vi "cRIO_4DOF_Admittance_control_v8c_eightmaze_MESO_removeIR.vi"() -> ()   [LabVIEW 2019]
uses:
  <vilib>/Platform/TimedLoop/XDataNode/timing_clust.ctl
  <vilib>/Platform/TimedLoop/XDataNode/nitl_modes.ctl
  <vilib>/Platform/TimedLoop/XDataNode/wakeup.ctl
  <vilib>/Analysis/baseanly.llb/Mean (DBL).vi
  Global 1.vi
  <vilib>/imath/engines/lvmath2/RunTimeEngine/NodeEndStatement/NIMS_NodeEndStatement_Output.vi
  <instcachedir>/0/NIMS_NodeEndStatement_Output_53EC0D466D134D7ABD903AC30B43404B.lvgen/NIMS_NodeEndStatement_Output_53EC0D466D134D7ABD903AC30B43404B_001.vi
  <vilib>/imath/engines/lvmath2/RunTimeEngine/ErrorHandling/NIMS_Finalize Error.vi
  <vilib>/imath/engines/lvmath2/RunTimeEngine/IndexReplace/NIMS V(S)=S.vi
  <instcachedir>/0/NIMS V(S)=S_BD5C8CB81B6E4D99B8C0034EA1BEE55D.lvgen/NIMS V(S)=S_BD5C8CB81B6E4D99B8C0034EA1BEE55D_000.vi
  <vilib>/imathl/engines/lvmath/Functions/Error Handling/Create Error.vi
  <instcachedir>/0/NIMS_NodeEndStatement_Output_53EC0D466D134D7ABD903AC30B43404B.lvgen/NIMS_NodeEndStatement_Output_53EC0D466D134D7ABD903AC30B43404B_005.vi
  <vilib>/addons/control/pid/pid.llb/PID (DBL Array).vi
  <vilib>/imath/engines/lvmath2/RunTimeEngine/ArithmeticOperatorToken/NIMS_ArithmeticOperator_multmx(M,CV).vi
  <instcachedir>/0/NIMS_ArithmeticOperator_multmx(M,CV)_1D61EED49E1847F3B05DBB8EDD2FBF8F.lvgen/NIMS_ArithmeticOperator_multmx(M,CV)_1D61EED49E1847F3B05DBB8EDD2FBF8F_000.vi
  <instcachedir>/0/NIMS_NodeEndStatement_Output_53EC0D466D134D7ABD903AC30B43404B.lvgen/NIMS_NodeEndStatement_Output_53EC0D466D134D7ABD903AC30B43404B_002.vi
  <vilib>/imath/engines/lvmath2/RunTimeEngine/BuiltInFunctions/inv/NIMS_inv(GM).vi
  <instcachedir>/0/NIMS_inv(GM)_A6DF8FE880224208AACFE4CF9F659502.lvgen/NIMS_inv(GM)_A6DF8FE880224208AACFE4CF9F659502_000.vi
  <vilib>/imath/engines/lvmath2/RunTimeEngine/ErrorHandling/NIMS_Create Error From Enums.vi
  <vilib>/imath/engines/lvmath2/RunTimeEngine/IndexRead/NIMS M(R2,S).vi
  <instcachedir>/0/NIMS M(R2,S)_56813DCFDD5A484292D2195AF15D2BF5.lvgen/NIMS M(R2,S)_56813DCFDD5A484292D2195AF15D2BF5_000.vi
  <vilib>/imath/engines/lvmath2/RunTimeEngine/IndexRead/NIMS M(S,S).vi
  <instcachedir>/0/NIMS M(S,S)_AC51E74150A542F7991B9634C66F3096.lvgen/NIMS M(S,S)_AC51E74150A542F7991B9634C66F3096_000.vi
  <vilib>/imath/engines/lvmath2/RunTimeEngine/Managers/WorkSpace/UID Generator.vi
  <vilib>/imath/engines/lvmath2/RunTimeEngine/BuiltInFunctions/round/NIMS_round(DBL-S).vi
  <vilib>/imath/engines/lvmath2/RunTimeEngine/IndexRead/NIMS V(S).vi
  <instcachedir>/0/NIMS V(S)_0488751826AF41519A22953C041130DC.lvgen/NIMS V(S)_0488751826AF41519A22953C041130DC_000.vi
  <vilib>/imath/engines/lvmath2/RunTimeEngine/RunTimeType/NIMS_RunTimeType_From StrictType (excl LVString).vi
  <instcachedir>/0/NIMS_RunTimeType_From StrictType (excl LVString)_D8AFBA86A94845AAA577C895450664BD.lvgen/NIMS_RunTimeType_From StrictType (excl LVString)_D8AFBA86A94845AAA577C895450664BD_000.vi
  <vilib>/imath/engines/lvmath2/RunTimeEngine/LocalVariableDefStatement/MC_LocalVariableDefStatement_Display.vi
  <vilib>/imath/engines/lvmath2/RunTimeEngine/BuiltInFunctions/all/NIMS_all(GS).vi
  <vilib>/imath/engines/lvmath2/RunTimeEngine/Managers/SymbolTable/Clear UID.vi
  <vilib>/imath/engines/lvmath2/RunTimeEngine/ArithmeticOperatorToken/NIMS_ArithmeticOperator_power(S).vi
  <instcachedir>/0/NIMS_ArithmeticOperator_power(S)_F1497A2DE3CE4E82B2C3646D59904248.lvgen/NIMS_ArithmeticOperator_power(S)_F1497A2DE3CE4E82B2C3646D59904248_014.vi
  <vilib>/imath/engines/lvmath2/RunTimeEngine/BuiltInFunctions/cross/NIMS_cross(GV,GV).vi
  <instcachedir>/0/NIMS_cross(GV,GV)_6F1F1C643EFF41C8A983D972A94A5A15.lvgen/NIMS_cross(GV,GV)_6F1F1C643EFF41C8A983D972A94A5A15_000.vi
  <vilib>/imath/engines/lvmath2/RunTimeEngine/IndexRead/NIMS M(S).vi
  <instcachedir>/0/NIMS M(S)_B826C018497E4940AE96BD27B540B6FB.lvgen/NIMS M(S)_B826C018497E4940AE96BD27B540B6FB_000.vi
  <vilib>/imath/engines/lvmath2/RunTimeEngine/BuiltInFunctions/norm/NIMS_norm(GM,DBL).vi
  <instcachedir>/0/NIMS_norm(GM,DBL)_8BCB088F207E48DF95CF5C1DC502F84D.lvgen/NIMS_norm(GM,DBL)_8BCB088F207E48DF95CF5C1DC502F84D_000.vi
  <vilib>/imath/engines/lvmath2/RunTimeEngine/BuiltInFunctions/norm/NIMS_norm(GV,DBL).vi
  <instcachedir>/0/NIMS_norm(GV,DBL)_4A8B6F23BC0A47549B8AB805006257D9.lvgen/NIMS_norm(GV,DBL)_4A8B6F23BC0A47549B8AB805006257D9_000.vi
  <vilib>/imath/engines/lvmath2/RunTimeEngine/BuiltInFunctions/dot/NIMS_dot(GM,GM,12).vi
  <instcachedir>/0/NIMS_dot(GM,GM,12)_05F0B1C82C6743E4843530F9B3085698.lvgen/NIMS_dot(GM,GM,12)_05F0B1C82C6743E4843530F9B3085698_000.vi
  <vilib>/imath/engines/lvmath2/RunTimeEngine/ArithmeticOperatorToken/NIMS_ArithmeticOperator_minus.vi
  <instcachedir>/0/NIMS_ArithmeticOperator_minus_12BFF9710EA5430A9EE87C5BC3F65186.lvgen/NIMS_ArithmeticOperator_minus_12BFF9710EA5430A9EE87C5BC3F65186_003.vi
  <vilib>/platform/TimedLoop/XDataNode/XDataNode.xnode
  <resource>/objmgr/ni.dex.rc
  <vilib>/addons/control/pid/NI_PID_pid.lvlib
  <vilib>/Analysis/NI_AALBase.lvlib
  <vilib>/Platform/TimedLoop/XDataNode/XDNodeRunTimeDep.lvlib
  <vilib>/imath/engines/lvmath2/RunTimeEngine/Managers/SymbolTable/NIMS_WorkSpace.lvlib
panel:
  in  "Global offset":dbl[](array[numeric])=[0.0, 0.0, 0.0, 0.0]
  in  "Half Dzone Limit":bool=TRUE
  in  "servo wait (ms)":u32=800
  in  "Servo enable":bool
  in  "No LEDs":bool=TRUE
  in  "Manual \npulse high":bool
  in  "cx start":dbl=1.0 format="%#_13g"
  in  "LED_R 2":bool
  in  "LED_L 2":bool
  in  "Flash LEDs":bool
  out "SynPulseOn":bool
  in  "RunOnceLatch":bool
  out "Data syncing":bool
  in  "No LED no Sound":bool
  in  "Mouse YStop":dbl=-0.33 format="%#_13g"
  out "Rmag":dbl
  out "w_cen 2":dbl[](array[numeric])
  out "Eight maze on":bool
  out "Loop_R Exit":bool
  out "Loop_L Exit":bool
  out "exit_pos":dbl[](array[numeric])
  out "Rexit":dbl
  out "exit_cen":dbl[](array[numeric])
  in  "End Wheel":bool
  in  "w_cen":dbl[](array[numeric])=[0.06, -0.2]
  in  "Rwheel":dbl=0.06
  in  "Begin Wheel":bool
  in  "delpos limits (+/-)\nadmittance control \nLoop":dbl[](array[numeric])=[0.0012, 0.0002, 0.0, 0.01]
  in  "delpos limits (+/-)\nadmittance control \nDzone":dbl[](array[numeric])=[0.0008, 0.0002, 0.0, 0.01]
  in  "Lego2":dbl=-0.03
  in  "Lego1":dbl=0.07
  in  "Ftrans":bool=TRUE
  out "TransF":dbl[](array[numeric])
  in  "d_{1}_{2} (mm)":dbl[](array[numeric])=[10.0, 0.0, 0.0]
  in  "MDsRy":dbl=0.251
  in  "MDsLy":dbl=-0.251
  out "MDsetup":bool
  in  "MDpos_lims":dbl[](array[numeric])=[0.0005, 0.0005]
  in  "MDstopR":dbl=0.025
  in  "Disable X":bool
  in  "MDstopL":dbl=0.023
  in  "Disable -X Dzone":bool
  in  "PWMset2":dbl[](array[numeric])=[8.1, 5.2, 5.45]
  in  "PWMset1":dbl[](array[numeric])=[3.4, 5.2, 5.45]
  in  "cMD":dbl=0.3 format="%#_13g"
  in  "mMD":dbl=0.02 format="%#_13g"
  in  "MDzone":dbl[](array[numeric])=[0.04, 0.027]
  out "Rsmall":dbl
  in  "Loop radius":dbl=0.127 format="%#_13g"
  in  "PWM positions":dbl[](array[numeric])=[4.5, 3.4, 5.1, 5.8]
  in  "PWM rate":dbl[](array[numeric])=[0.1, 0.1, 0.1, 0.1]
  out "appended array":bool[](array[boolean])
  in  "LED_L":bool
  in  "LED_R":bool
  in  "MD_L":bool
  in  "MD_R":bool
  out "Left":bool=TRUE
  in  "AIR":bool
  in  "Sound":bool
  out "Right":bool=TRUE
  in  "MD time (ms)":i32=4000
  in  "Loop seq.":dbl
  in  "Initialize":bool=TRUE
  in  "No Milk":bool
  out "All BBL":bool
  out "BB3_L":bool
  out "BB2_L":bool
  out "BB1_R":bool
  out "All BBR":bool
  out "BB3_R":bool
  out "BB2_R":bool
  out "BB1_L":bool
  out "Seq update":i32
  in  "Repeat sound":bool
  in  "Air puff time":u32=1000
  out "Direction array":bool[](array[boolean])=[TRUE, FALSE, FALSE, TRUE, FALSE, TRUE, TRUE, FALSE, TRUE, FALSE, FALSE, TRUE, FALSE, TRUE, FALSE, FALSE, TRUE, FALSE, TRUE, TRUE, FALSE, TRUE, FALSE, FALSE, TRUE, FALSE, TRUE, TRUE, FALSE, TRUE, FALSE, FALSE, TRUE, FALSE, TRUE, TRUE, FALSE, TRUE, FALSE, FALSE, TRUE, FALSE, TRUE, TRUE, FALSE, TRUE, FALSE, FALSE, TRUE]
  in  "cTrans":dbl=0.01 format="%#_13g"
  out "C":dbl
  out "Dzone y 2":dbl=-0.0607 format="%#_13g"
  in  "Vector correction":bool=TRUE
  in  "manual homing stop":bool
  in  "cLoop":dbl=0.3
  in  "mLoop":dbl=0.02
  out "c_applied":dbl[][](array[numeric])
  out "m_applied":dbl[][](array[numeric])
  in  "lower Z limit":dbl=-0.782
  out "Jostick offset":dbl[](array[numeric])
  out "Pos":dbl[](array[numeric])
  out "targetpos":dbl[](array[numeric])
  out "Rotz":dbl[][](array[numeric])
  in  "Eight maze on":bool
  out "Gradient R":dbl=0.0293 format="%#_13g"
  out "Radius":dbl=0.0293 format="%#_13g"
  out "Dzone y":dbl=0.025 format="%#_13g"
  out "Loop_L":bool
  out "F":dbl[](array[numeric])
  in  "number Fsamples":i32=10
  out "Homed":bool[](array[boolean])
  out "Hall voltages":dbl[](array[numeric])
  in  "Joint offset":dbl[](array[numeric])
  in  "Target HallV":dbl[](array[numeric])=[0.1, 0.1, 0.1]
  out "Raw voltages":dbl[](array[numeric])
  in  "Record to current file":bool
  in  "Close file and open new file":bool
  in  "Stop raspberry pi":bool
  out "changes from \nadmittance {m}":dbl[](array[numeric])
  out "Joystick input":dbl[](array[numeric])
  in  "Joystick control on":bool
  out "Z position":T1(graph)
  out "Loop_R":bool
  out "Trajectory changes in Yaw":T1(graph)
  in  "Mouse force limits":dbl[](array[numeric])=[0.5, 0.2, 0.0, 0.025]
  out "loop":i32
  in  "Disable Yaw forces":bool=TRUE
  in  "Admittance scale":dbl[](array[numeric])=[1.0, 1.0, 0.0, 1.0]
  out "velocity \n(mouseframe)":dbl[](array[numeric])
  in  "RETURN TO HOME \nPOSITION AND STOP":bool
  out "Dzone":bool
  in  "deltapos":dbl[](array[numeric]) format="%#_13g"
  in  "delpos limits (+/-) \ntrajectory control\n(global frame)":dbl[](array[numeric])=[0.002, 0.002, 0.0, 0.02]
  in  "delpos limits (+/-)\nadmittance control \n(mouse frame)":dbl[](array[numeric])=[0.0015, 0.0002, 0.0, 0.01]
  in  "lower limit":dbl[](array[numeric])=[-0.3, -0.34, -0.782, -6000.0]
  in  "upper limit":dbl[](array[numeric])=[0.3, 0.18, -0.65, 6000.0]
  out "Dzone x":dbl=-0.0607 format="%#_13g"
  in  "Trajectory scale":dbl[](array[numeric])=[0.05, 0.05, 0.0, 0.05]
  out "Trajectory changes in XY":T1(graph)
  in  "Disable Y forces":bool=TRUE
  out "changes from trajectory":dbl[](array[numeric])
  in  "Y_trajectory":bool
  in  "Disable -X":bool=TRUE
  out "Eightmaze_switch":bool
  in  "Yaw":dbl(slide) scale=0.0..3.142
  in  "Z":dbl(slide)=-0.7034810126582278 scale=-0.1..0.1
  in  "Y":dbl(slide)=0.05 scale=-0.29..0.05
  in  "X":dbl(slide) scale=0.0..0.06
  in  "Yaw_tajectory":bool
  out "target position":dbl[](array[numeric])
  in  "Fsense deadband\n (Nm or N)":dbl[](array[numeric])=[0.025, 0.025, 0.025, 0.001]
  in  "Output range (PWM)":cluster{"output high":dbl, "output low":dbl}[](array[cluster])=[{"output high"=100.0, "output low"=-100.0}] {"output low" format="%.2f"; "output high" format="%.2f"}
  in  "Admittance PID gains":T2(array[cluster])=[{"proportional gain (Kc)"=1.0, "integral time (Ti, min)"=0.01, "derivative time (Td, min)"=0.0}] {"derivative time (Td, min)" format="%.3f"; "integral time (Ti, min)" format="%.3f"; "proportional gain (Kc)" format="%.3f"}
  in  "Manual force":bool
  in  "Manual forces\n(mouse frame)":dbl[](array[numeric])=[0.0, 0.0, 0.0, 0.0, 0.0, 0.0]
  in  "goniometer PWM\n offset":dbl=50.0
  in  "delta PWM offset":dbl[](array[numeric])=[50.0, 50.0, 50.0]
  in  "manual position\n(global frame)":dbl[](array[numeric])=[0.0, 0.0, 0.0, 0.0, 0.0, 0.0]
  in  "Manual position control":bool
  out "Forces (N) 2":T3(graph)
  out "Torques (Nm) 2":T3(graph)
  in  "Measure Fsensor \nV offset":bool
  out "Sensor V offset":dbl[](array[numeric])
  out "Mouse forces":dbl[](array[numeric])
  in  "Out of range":bool
  out "F_measured":dbl[](array[numeric])
  out "velocity\n(global frame)":dbl[](array[numeric])
  out "Admittance changes in Yaw":T3(graph)
  out "Admittance changes in XY":T3(graph)
  out "Torques (Nm)":T3(graph)
  out "Forces (N)":T3(graph)
  in  "m":dbl[][](array[numeric])=[[0.02, 0.0, 0.0, 0.0], [0.0, 0.02, 0.0, 0.0], [0.0, 0.0, 0.30000000000000004, 0.0], [0.0, 0.0, 0.0, 2e-05]]
  in  "c":dbl[][](array[numeric])=[[0.5, 0.0, 0.0, 0.0], [0.0, 0.2, 0.0, 0.0], [0.0, 0.0, 2.0, 0.0], [0.0, 0.0, 0.0, 0.0002]]
  out "True loop time (ms)":u32
  in  "theta6":dbl
  in  "theta1,2,3 pos2":dbl=-0.75
  in  "Initial pos 2":bool
  in  "Theta PID gains":T2(array[cluster])=[{"proportional gain (Kc)"=1.0, "integral time (Ti, min)"=0.01, "derivative time (Td, min)"=0.0}] {"derivative time (Td, min)" format="%.3f"; "integral time (Ti, min)" format="%.3f"; "proportional gain (Kc)" format="%.3f"}
  in  "Theta output range":cluster{"output high":dbl, "output low":dbl}[](array[cluster])=[{"output high"=100.0, "output low"=-100.0}] {"output low" format="%.2f"; "output high" format="%.2f"}
  in  "theta 6":dbl
  in  "theta1,2,3":dbl=-0.75
  in  "Stop Joint space control":bool
  in  "Disable PID":bool
  out "velocity \n(joint space)":dbl[](array[numeric])
  out "op-space pos\n(global frame)":dbl[](array[numeric])
  out "alpha beta gamma":T1(graph)
  out "PWM":T4(graph)
  out "XY position":T1(graph)
  out "discriminant (>0)":dbl
  in  "Loop time (ms)":i64=10
  out "Data output":dbl[][](array[numeric])
  out "network stream":errorcluster
  out "Available Elements for Writing in network stream":i32
  in  "STOP saving data set":bool
  in  "PAUSE ms to wait":u32=5000
  in  "PAUSE saving data set":bool
  in  "BEGIN saving new data set":bool
  out "J":dbl[][](array[numeric])
  out "Joint_pos (rad)":dbl[](array[numeric])
  # "VALUE USED FOR INITIALISATION, TROUBLESHOOTING AND ANALYSIS"
  # "Must start USB6211DAQ.vi to read voltages from force sensor"
  # "Data saving. 'Write data to tdms file (PC VI).vi' must be started\n BEFORE this vi in order for the network stream to open correctly.\nMake sure 'Write data to tdms file (PC VI).vi' is configured correctly"
  # "Initialise system; both buttons must be pressed sequentially, left then right. Press Stop JSC when AB offset = Joint_pos"
  # "STOP AND RETURN TO HOME"
  # "VELOCITY LIMITS NB: delpos*100 = max velocity"
  # "Trajectory control. Push these buttons after manually moving the headstage to X,Y=0 m, yaw = 3.142 rad"
  # "Use Manual position control to set up or adjust the headstage position; the sliders ADD ON to the current position."
  # "POSITION LIMITS"
  # "NB: if True loop time does not equal Loop time\nthen the virtual admittance will not be correct"
  # "Admittance control. Manual position control must be switched OFF for Admittance control to work."
  # "Trajectory parameters"
  # "8 maze controls - air puff manually activated; 3000ms MD time = 8uL milk"
  # "IR camera control: record should \nremain on while recording; close \nfile and open new for each mouse"
  # "Rdown"
  # "Lup"
  # "Rup"
  # "Ldown"
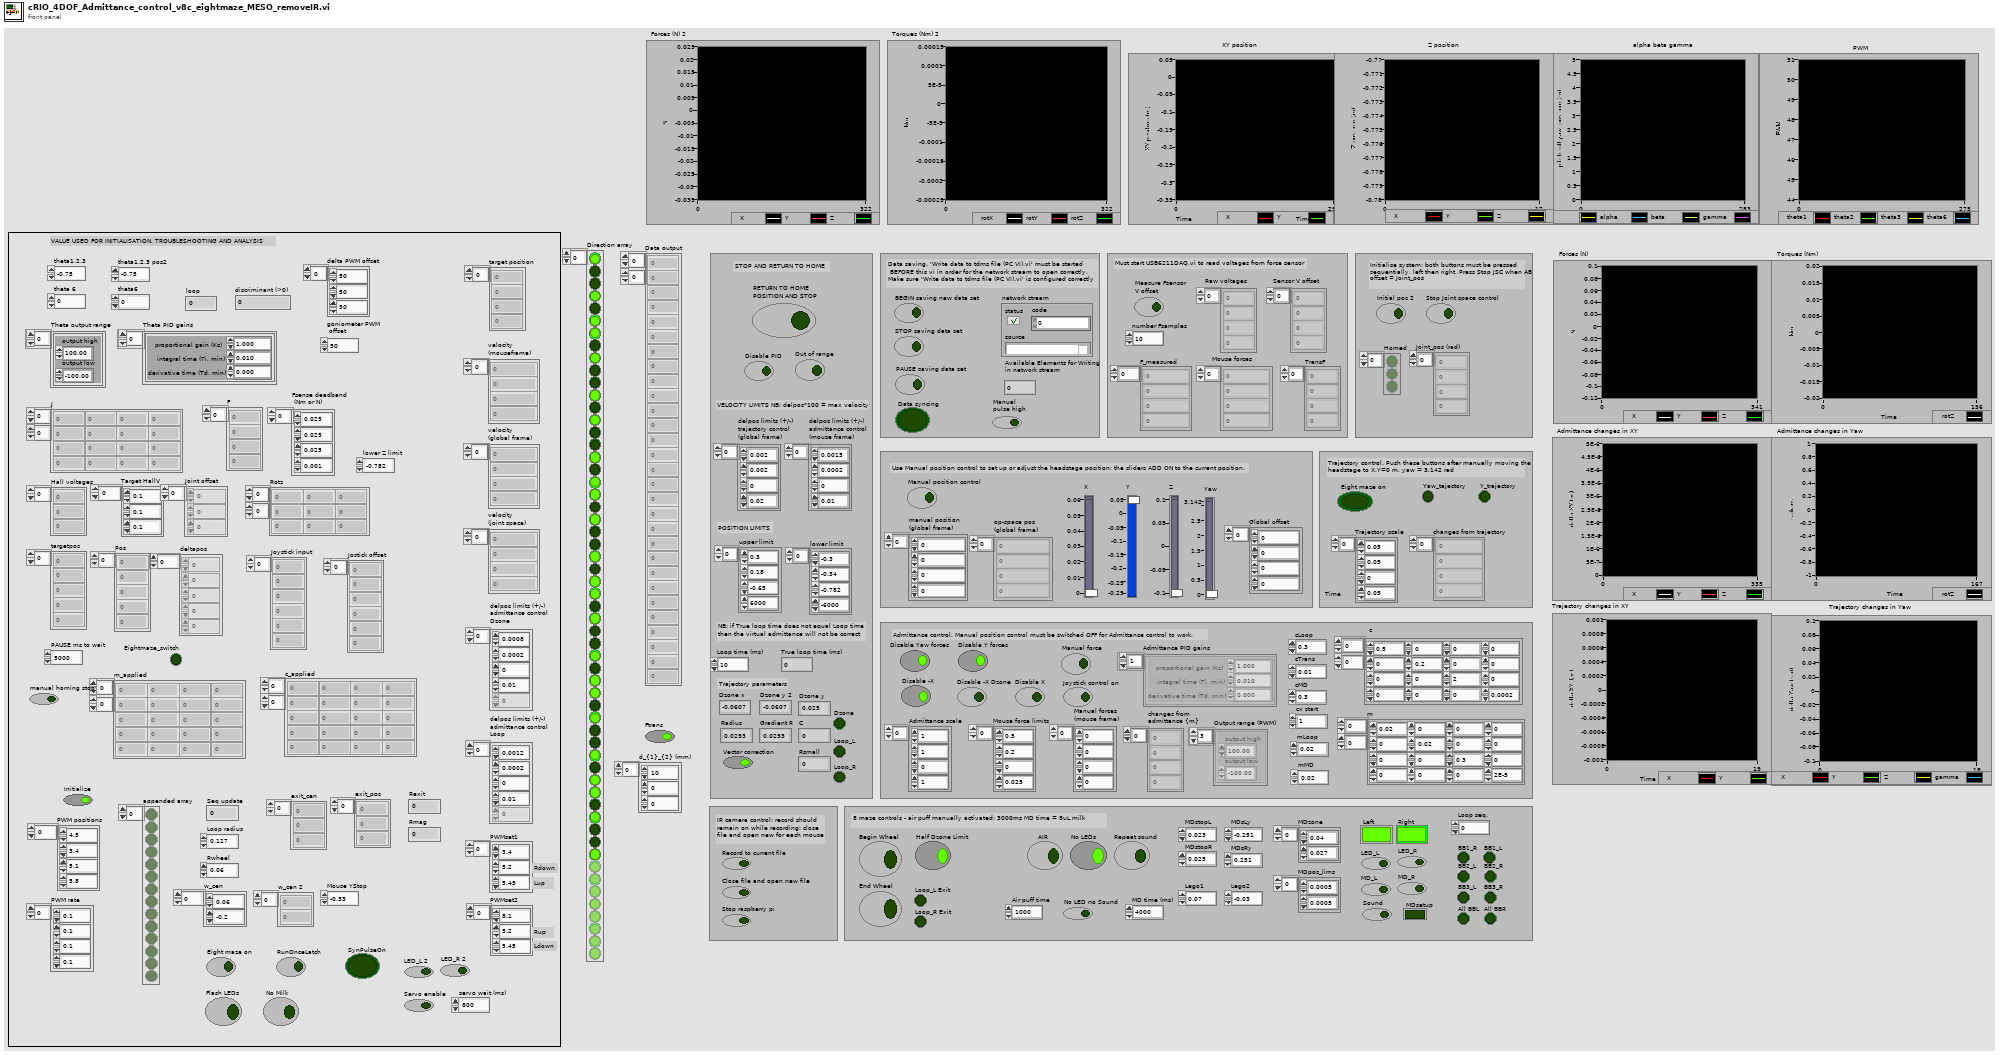
[diagram p1: front panel]
types:
  T1 = cluster{"Joint_pos (rad)[0]":dbl, "Joint_pos (rad)[1]":dbl, "Joint_pos (rad)[2]":dbl, "Joint_pos (rad)[3]":dbl, "Joint_pos (rad)[4]":dbl, "Joint_pos (rad)[5]":dbl, "Joint_pos (rad)[6]":dbl, "Joint_pos (rad)[7]":dbl, "Joint_pos (rad)[8]":dbl}
  T2 = cluster{"proportional gain (Kc)":dbl, "integral time (Ti, min)":dbl, "derivative time (Td, min)":dbl}[]
  T3 = cluster{"F[0]":dbl, "F[1]":dbl, "F[2]":dbl, "F[3]":dbl, "F[4]":dbl, "F[5]":dbl, "F[6]":dbl, "F[7]":dbl, "F[8]":dbl}
  T4 = cluster{"[0]":dbl, "[1]":dbl, "[2]":dbl, "[3]":dbl, "[4]":dbl, "[5]":dbl, "[6]":dbl, "[7]":dbl, "[8]":dbl}
  T5 = typedef "XDNodeRunTimeDep.lvlib/timing_clust.ctl" = cluster{"Expected End [f-1]":u64, "Actual End [f-1]":u64, "Finished Late? [f-1]":bool, "Expected End [i-1]":u64, "Actual End [i-1]":u64, "Finished Late? [i-1]":bool, "Expected Start [i]":u64, "Actual Start [i]":u64, "Expected Start [f]":u64, "Actual Start [f]":u64, "Source Name":string, "Structure Name":string, "Period":i64, "Deadline":i64, "Offset":i64, "Start":i64, "Priority":i32, "Timeout":i32, "Mode":T6, "Wakeup Reason":T7, "Error":errorcluster, "Source Type":string, "Secondary Source Type":string, "Global End Time":u64, "Global Start Time":u64, "Frame Duration":u64, "Iteration Duration":u64, "Assigned CPU":i32, "I/O Scan Engine Mode":u32}
  T6 = typedef "XDNodeRunTimeDep.lvlib/nitl_modes.ctl" = enum32{"No Change", "Process missed periods, maintain original phase", "Discard missed periods, maintain original phase", "Process missed periods, ignore original phase", "Discard missed periods, ignore original phase"}
  T7 = typedef "XDNodeRunTimeDep.lvlib/wakeup.ctl" = enum32{"Normal", "Aborted", "Asynchronous wakeup", "Timing source error", "Timed loop error", "Timeout"}
  T8 = cluster{"op-space pos\n(global frame)[0]":dbl, "op-space pos\n(global frame)[1]":dbl, "op-space pos\n(global frame)[2]":dbl, "op-space pos\n(global frame)[3]":dbl, "op-space pos\n(global frame)[4]":dbl, "op-space pos\n(global frame)[5]":dbl, "op-space pos\n(global frame)[6]":dbl, "op-space pos\n(global frame)[7]":dbl, "op-space pos\n(global frame)[8]":dbl}
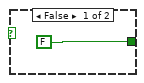
[diagram p3: hidden frame]
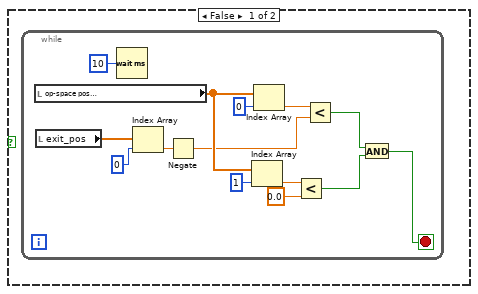
[diagram p4: hidden frame]
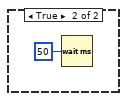
[diagram p5: hidden frame]
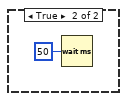
[diagram p6: hidden frame]
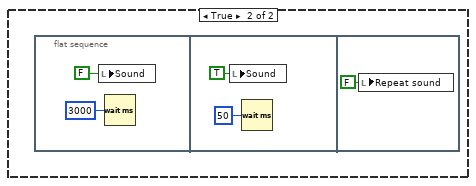
[diagram p8: hidden frame]
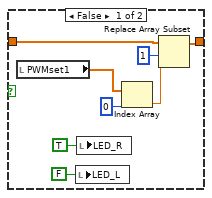
[diagram p9: hidden frame]
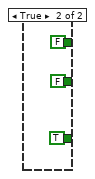
[diagram p12: hidden frame]
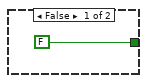
[diagram p14: hidden frame]
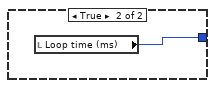
[diagram p16: hidden frame]
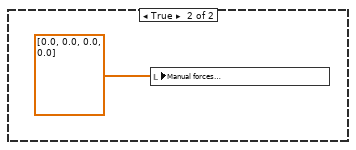
[diagram p17: hidden frame]
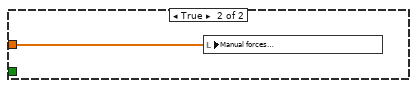
[diagram p18: hidden frame]
diagram:
  n1 = flat-sequence {
    frame #0 {
      n2 = local write "RunOnceLatch"(TRUE ("RunOnceLatch")) -> ()
    }
    frame #1 {
      n3 = while {
        stop <- FALSE stop-if-true
        n4 = flat-sequence {
          frame #0 {
            n5 = while {
              stop <- w10 stop-if-true
              n6 = local read "Eight maze on"() -> (w9:bool)
              n7 = local read "Begin Wheel"() -> (w7:bool)
              n8 = Not(x=w9) -> (.not. x?=w8:bool)
              n9 = Wait (ms)(milliseconds to wait=u32 250) -> ()  [unwired: 1 out]
              n10 = Compound Arithmetic op=AND(w7, w8, "RunOnceLatch") -> (w10:bool)
            }
          }
          frame #1 {
            n11 = disable-structure shown="Disabled" {
              frame Disabled {
                n12 = while {
                  stop <- w14 stop-if-true
                  n13 = local read "op-space pos\n(global frame)"() -> (w24:dbl[])
                  n14 = Wait (ms)(milliseconds to wait=u32 10) -> ()  [unwired: 1 out]
                  n15 = local read "w_cen"() -> (w21:dbl[])
                  n16 = Index Array(array=w21, index=0) -> (element=w19:dbl)
                  n17 = Index Array(array=w21, index=1) -> (element=w17:dbl)
                  n18 = Index Array(array=w24, index=0) -> (element=w20:dbl)
                  n19 = Index Array(array=w24, index=1) -> (element=w18:dbl)
                  n20 = local read "op-space pos\n(global frame)"() -> (w28:dbl[])
                  n21 = mathscript code="xpos = Pos(1,1);\nypos = Pos(1,2);\nzpos = Pos(1,3);\nyawpos = Pos(1,4);\n\nRotz = [cos(yawpos),-sin(yawpos),0; sin(yawpos),cos(yawpos),0; 0,0,1];\nxhat = [1, 0, 0]';\nzhat = [0, 0, 1]';\n\n       xcen = xpos - w_cen(1);\n       ycen = ypos - w_cen(2);\n       Rmag = real((xcen^2 + ycen^2)^0.5);\n       xtarg = Rwheel/Rmag*xcen  + w_cen(1);\n       ytarg = Rwheel/Rmag*ycen + w_cen(2);      \n       RLsgn = 1;\n\nvecpos = [xcen, ycen, 0]';         % position vector, zero'd circle\nvecyaw = RLsgn*cross(vecpos,zhat);  % yaw vector\nvecyaw_o = Rotz'*vecyaw;        %  yaw vector transformed by actual yaw\nyawerrsign = sign(0 - vecyaw_o(2));  % sign of yaw error\nyawerrmag = acos(dot(vecyaw_o,xhat)/(norm(vecyaw_o)*norm(xhat))); % magnitude of yaw error   \nyawtarg  = yawpos - yawerrsign*real(yawerrmag); % target yaw position\n\ntargetpos = [xtarg, ytarg, zpos, yawtarg];\n\ndelpos = real(targetpos - Pos);"("Pos"=w28, "Rwheel"="Rwheel", "w_cen"="w_cen") -> ("delpos"=w12:dbl[])  [unwired: 1 in, 1 out]
                  n22 = Less?(x=w20, y=w19) -> (x < y?=w16:bool)
                  n23 = Greater?(x=w18, y=w17) -> (0:w15:bool)
                  n24 = And(x=w16, y=w15) -> (x .and. y?=w14:bool)
                  n25 = local write "deltapos"(w12) -> ()
                }
              }
              frame Enabled {
              }
            }
          }
          frame #2 {
            n26 = local read "op-space pos\n(global frame)"() -> (w441:dbl[])
            n27 = Index Array(array=w441, index=3) -> (element=w442:dbl)
            n28 = while {
              tunnel: w442 -> [w457]
              stop <- w450 stop-if-true
              n29 = local read "op-space pos\n(global frame)"() -> (w456:dbl[])
              n30 = local read "w_cen"() -> (w455:dbl[])
              n31 = local write "Disable Yaw forces"(TRUE ("Disable Yaw forces")) -> ()
              n32 = local write "Disable Y forces"(TRUE ("Disable Y forces")) -> ()
              n33 = mathscript code="xpos = Pos(1,1);\nypos = Pos(1,2);\nzpos = Pos(1,3);\nyawpos = Pos(1,4);\n\nxtarg = 0;\nyawtarg = pi/2;\n\ntargetpos = [xtarg, ypos, zpos, yawtarg];\n\ndelpos = real(targetpos - Pos);"("yaw_init"=w457, "Pos"=w456, "w_cen"=w455) -> ("delpos"=w449:dbl[])  [unwired: 1 in, 1 out]
              n34 = local write "Disable -X"(TRUE ("Disable -X")) -> ()
              n35 = local write "delpos limits (+/-)\nadmittance control \n(mouse frame)"(dbl[] [0.0008, 0.0002, 0.0, 0.01] ("delpos limits (+/-)\nadmittance control \nDzone")) -> ()
              n36 = local read "op-space pos\n(global frame)"() -> (w453:dbl[])
              n37 = Index Array(array=w453, index=1) -> (element=w452:dbl)
              n38 = local write "deltapos"(w449) -> ()
              n39 = Greater?(x=w452, y=0.0) -> (0:w450:bool)
              n40 = Wait (ms)(milliseconds to wait=u32 10) -> ()  [unwired: 1 out]
            }
          }
          frame #3 {
            n41 = local write "RunOnceLatch"(FALSE ("RunOnceLatch")) -> ()
            n42 = local write "Eight maze on"(TRUE ("Eight maze on")) -> ()
            n43 = local write "Begin Wheel"(FALSE ("Begin Wheel")) -> ()
          }
        }
      }
    }
  }
  n44 = flat-sequence {
    frame #0 {
      w614 = -0.02 ("Dzone x")
      w628 = 0.0 ("X")
      n45 = mathscript code="Dx = R - R*cos(pi/4);\nDy = R*sin(pi/4);\n\nGrad_R = -Dx/Dy;\n\nh = R/cos(pi/4);\n\nRsmall = h - R;"("R"="Loop radius") -> ("Dx"=→"Dzone x":dbl, "Dy"=→"Dzone y":dbl, "Grad_R"=w609:dbl, "Rsmall"=→"Rsmall":dbl)  [unwired: 1 in, 1 out]
      "Gradient R" <- w609
      n46 = mathscript code="x1 = R*cos(pi/4) + -R;\n\nRexit = x1/(cos(pi*3/4) - 1);\n\nexit_cen(1) = -Rexit;\n\ny1 = -R*sin(pi/4) + 0;\n\nexit_cen(2) = y1 - Rexit*sin(pi*3/4);\n\nexit_pos = [x1, y1];"("R"="Loop radius") -> ("exit_cen"=→"exit_cen":dbl[], "Rexit"=→"Rexit":dbl, "exit_pos"=→"exit_pos":dbl[])  [unwired: 1 in, 1 out]
      n47 = local write "RETURN TO HOME \nPOSITION AND STOP"(FALSE ("RETURN TO HOME \nPOSITION AND STOP")) -> ()
      n48 = local write "Joystick control on"(FALSE ("Joystick control on")) -> ()
      n49 = local write "Initial pos 2"(FALSE ("Initial pos 2")) -> ()
      n50 = local write "Stop Joint space control"(FALSE ("Stop Joint space control")) -> ()
      n51 = local write "Disable PID"(TRUE ("Disable PID")) -> ()
      n52 = local write "Manual force"(FALSE ("Manual force")) -> ()
      n53 = local write "Manual \npulse high"(FALSE ("Manual pulse high")) -> ()
      n54 = local write "Half Dzone Limit"(TRUE ("Half Dzone Limit")) -> ()
      n55 = local write "Manual position control"(TRUE ("Manual velocity control")) -> ()
      n56 = local write "Begin Wheel"(FALSE ("Begin Wheel")) -> ()
      n57 = local write "Disable PID"(FALSE ("Enable PID")) -> ()
      n58 = local write "Yaw_tajectory"(FALSE ("Mousetrack_Yaw")) -> ()
      n59 = local write "Y_trajectory"(FALSE ("Mousetrack_Yaw")) -> ()
      n60 = local write "Eight maze on"(FALSE ("Trajectory control")) -> ()
      n61 = shared-variable "RT CompactRIO Target\\Mod7\\DIO0"(FALSE ("DIO0")) -> ()  [unwired: 1 in, 1 out]
      n62 = local write "theta1,2,3 pos2"(-0.25 ("theta1,2,3 pos2")) -> ()
      n63 = local write "theta1,2,3"(-0.75 ("theta1,2,3")) -> ()
      n64 = global write "Global 1.vi" "a_1 (m)"(0.1 ("a_4 (m)")) -> ()
      n65 = local write "Manual forces\n(mouse frame)"(dbl[] [0.0, 0.0, 0.0, 0.0] ("Manual forces")) -> ()
      n66 = local write "Yaw"(w628) -> ()
      n67 = local write "theta6"(0.0 ("theta4,5,6")) -> ()
      n68 = global write "Global 1.vi" "Rf (m)"(0.1898 ("Rf (m)")) -> ()
      n69 = global write "Global 1.vi" "Ld (m)"(0.656 ("Ld (m)")) -> ()
      n70 = global write "Global 1.vi" "L6 (m)"(0.22 ("a_4 (m)")) -> ()
      n71 = global write "Global 1.vi" "Rm (m)"(0.1 ("Rm (m)")) -> ()
      n72 = global write "Global 1.vi" "Lp (m)"(0.34 ("Lp (m)")) -> ()
      n73 = local write "Y"(w628) -> ()
      n74 = local write "X"(w628) -> ()
      n75 = local write "Z"(w628) -> ()
      n76 = local write "Close file and open new file"(FALSE ("Close file and open new file")) -> ()
      n77 = local write "Record to current file"(FALSE ("Record to current file")) -> ()
      n78 = Multiply(x=w609, y=w614) -> (x*y=w613:dbl)
      n79 = local write "Stop raspberry pi"(FALSE ("Stop raspberry pi")) -> ()
      n80 = Negate(x=w613) -> (-x=→"C":dbl)
      n81 = local write "Target HallV"(dbl[] [0.1, 0.1, 0.1] ("Joint offset")) -> ()
      n82 = local write "Theta output range"(cluster{"output high":dbl, "output low":dbl}[] [{"output high"=50.0, "output low"=-50.0}] ("XYZ output range")) -> ()
      n83 = local write "Theta PID gains"(T2 [{"proportional gain (Kc)"=10.0, "integral time (Ti, min)"=0.0, "derivative time (Td, min)"=0.0}] ("XYZ PID gains")) -> ()
      n84 = local write "Admittance PID gains"(T2 [{"proportional gain (Kc)"=80.0, "integral time (Ti, min)"=0.5, "derivative time (Td, min)"=0.0}, {"proportional gain (Kc)"=80.0, "integral time (Ti, min)"=0.5, "derivative time (Td, min)"=0.0}, {"proportional gain (Kc)"=40.0, "integral time (Ti, min)"=0.5, "derivative time (Td, min)"=0.0}, {"proportional gain (Kc)"=200.0, "integral time (Ti, min)"=0.0, "derivative time (Td, min)"=0.0}] ("XYZ PID gains")) -> ()
      n85 = local write "Output range (PWM)"(cluster{"output high":dbl, "output low":dbl}[] [{"output high"=50.0, "output low"=-50.0}, {"output high"=50.0, "output low"=-50.0}, {"output high"=50.0, "output low"=-50.0}, {"output high"=50.0, "output low"=-50.0}] ("XYZ output range")) -> ()
      n86 = local write "upper limit"(dbl[] [0.3, 0.18, -0.65, 6000.0] ("upper limit")) -> ()
      n87 = local write "lower limit"(dbl[] [-0.3, -0.34, -0.782, -6000.0] ("lower limit")) -> ()
      "Radius" <- "Loop radius"
      "Dzone y 2" <- w614
    }
    frame #1 {
      n88 = while {
        stop <- w830 stop-if-true
        w840 = dbl[] [50.0, 50.0, 50.0]  # PWM 50% offset
        n89 = shared-variable "RT CompactRIO Target\\Mod8\\AI28"() -> (w848:dbl)  [unwired: 1 in, 1 out]
        n90 = shared-variable "RT CompactRIO Target\\Mod8\\AI27"() -> (w847:dbl)  [unwired: 1 in, 1 out]
        n91 = shared-variable "RT CompactRIO Target\\Mod8\\AI20"() -> (w849:dbl)  [unwired: 1 in, 1 out]
        n92 = Build Array(w849, w848, w847) -> (w836:dbl[])
        "Hall voltages" <- w836
        n93 = call-poly <vilib>:"PID.vi"("output range"=cluster{"output high":dbl, "output low":dbl}[] [{"output high"=5.0, "output low"=-5.0}], "PID gains"=T2 [{"proportional gain (Kc)"=4.0, "integral time (Ti, min)"=0.0, "derivative time (Td, min)"=0.0}], "process variable"=w836, "setpoint"="Target HallV") -> ("output"=w833:dbl[])  [unwired: 6 in, 1 out]
        n94 = Negate(x=w833) -> (-x=w832:dbl[])
        n95 = Add(x=w832, y=w840) -> (x+y=w839:dbl[])
        n96 = Add(x=dbl[] [0.05, 0.05, 0.05], y="Target HallV") -> (x+y=w835:dbl[])
        n97 = Subtract(x="Target HallV", y=dbl[] [0.0, 0.0, 0.0]) -> (x-y=w826:dbl[])
        n98 = Index Array(array=w839, index=1) -> (element=w842:dbl)
        n99 = Index Array(array=w839, index=0) -> (element=w843:dbl)
        n100 = Index Array(array=w839, index=2) -> (element=w841:dbl)
        n101 = In Range and Coerce(upper limit=w835, x=w836, lower limit=w826) -> (In Range?=w834:bool[])  [unwired: 1 out]
        "Homed" <- w834
        n102 = And Array Elements(Boolean array=w834) -> (logical AND=w831:bool)
        n103 = In Range and Coerce(upper limit=52.0, x=w843, lower limit=48.0) -> (coerced(x)=w852:dbl)  [unwired: 1 out]
        n104 = In Range and Coerce(upper limit=52.0, x=w842, lower limit=48.0) -> (coerced(x)=w851:dbl)  [unwired: 1 out]
        n105 = In Range and Coerce(upper limit=52.0, x=w841, lower limit=48.0) -> (coerced(x)=w850:dbl)  [unwired: 1 out]
        n106 = Or(x=w831, y="manual homing stop") -> (x .or. y?=w830:bool)
        n107 = shared-variable "RT CompactRIO Target\\Mod5\\PWM1"(w851) -> ()  [unwired: 1 in, 1 out]
        n108 = shared-variable "RT CompactRIO Target\\Mod5\\PWM2"(w850) -> ()  [unwired: 1 in, 1 out]
        n109 = shared-variable "RT CompactRIO Target\\Mod5\\PWM0"(w852) -> ()  [unwired: 1 in, 1 out]
      }
    }
    frame #2 {
      n110 = call "cRIO_4DoF_Encoders_counts2rad(subVI).vi"() -> ("Theta3"=w860:dbl, "Theta2"=w861:dbl, "Theta1"=w862:dbl, "Theta6"=w863:dbl)  [unwired: 4 in]
      n111 = Build Array(w862, w861, w860, w863) -> (w859:dbl[])
      n112 = local write "Joint offset"(w859) -> ()
    }
    frame #3 {
      n113 = while "Joint space control" {
        stop <- w871 stop-if-true
        w874 = dbl[] [50.0, 50.0, 50.0, 50.0]  # PWM 50% offset
        n114 = case shown="False" "Initial pos 2" {
          tunnel: [w896 w897] -> w891
          frame False {
            n115 = Build Array("theta1,2,3", "theta1,2,3", "theta1,2,3", "theta 6") -> (w896:dbl[])
          }
          frame True {
            n116 = Build Array("theta1,2,3 pos2", "theta1,2,3 pos2", "theta1,2,3 pos2", "theta6") -> (w897:dbl[])
          }
        }
        n117 = local read "Joint_pos (rad)"() -> (w865:dbl[])
        n118 = call-poly <vilib>:"PID.vi"("output range"="Theta output range", "PID gains"="Theta PID gains", "process variable"=w865, "setpoint"=w891) -> ("output"=w864:dbl[])  [unwired: 6 in, 1 out]
        n119 = Add(x=w864, y=w874) -> (x+y=w873:dbl[])
        n120 = Index Array(array=w873, index=0) -> (element=w886:dbl)
        n121 = Index Array(array=w873, index=1) -> (element=w877:dbl)
        n122 = Index Array(array=w873, index=2) -> (element=w876:dbl)
        n123 = Index Array(array=w873, index=3) -> (element=w875:dbl)
        n124 = In Range and Coerce(upper limit=99.0, x=w886, lower limit=1.0) -> (coerced(x)=w869:dbl)  [unwired: 1 out]
        n125 = In Range and Coerce(upper limit=99.0, x=w877, lower limit=1.0) -> (coerced(x)=w868:dbl)  [unwired: 1 out]
        n126 = In Range and Coerce(upper limit=99.0, x=w875, lower limit=1.0) -> (coerced(x)=w866:dbl)  [unwired: 1 out]
        n127 = In Range and Coerce(upper limit=99.0, x=w876, lower limit=1.0) -> (coerced(x)=w867:dbl)  [unwired: 1 out]
        n128 = shared-variable "RT CompactRIO Target\\Mod5\\PWM2"(w867) -> ()  [unwired: 1 in, 1 out]
        n129 = shared-variable "RT CompactRIO Target\\Mod5\\PWM3"(w866) -> ()  [unwired: 1 in, 1 out]
        n130 = shared-variable "RT CompactRIO Target\\Mod5\\PWM0"(w869) -> ()  [unwired: 1 in, 1 out]
        n131 = shared-variable "RT CompactRIO Target\\Mod5\\PWM1"(w868) -> ()  [unwired: 1 in, 1 out]
        n132 = And(x="Stop Joint space control", y="Initial pos 2") -> (x .and. y?=w871:bool)
      }
    }
    frame #4 {
      w916 = dbl[] [50.0, 50.0, 50.0, 50.0] ("y")
      w922 = 0.0 ("X")
      n133 = Wait (ms)(milliseconds to wait=u32 50) -> ()  [unwired: 1 out]
      n134 = Index Array(array=w916, index=0) -> (element=w903:dbl)
      n135 = Index Array(array=w916, index=1) -> (element=w902:dbl)
      n136 = Index Array(array=w916, index=2) -> (element=w901:dbl)
      n137 = Index Array(array=w916, index=3) -> (element=w900:dbl)
      n138 = local write "Yaw"(w922) -> ()
      n139 = local write "Z"(w922) -> ()
      n140 = local write "Y"(w922) -> ()
      n141 = In Range and Coerce(upper limit=99.0, x=w903, lower limit=1.0) -> (coerced(x)=w907:dbl)  [unwired: 1 out]
      n142 = local write "X"(w922) -> ()
      n143 = In Range and Coerce(upper limit=99.0, x=w902, lower limit=1.0) -> (coerced(x)=w906:dbl)  [unwired: 1 out]
      n144 = In Range and Coerce(upper limit=99.0, x=w901, lower limit=1.0) -> (coerced(x)=w905:dbl)  [unwired: 1 out]
      n145 = In Range and Coerce(upper limit=99.0, x=w900, lower limit=1.0) -> (coerced(x)=w904:dbl)  [unwired: 1 out]
      n146 = shared-variable "RT CompactRIO Target\\Mod5\\PWM0"(w907) -> ()  [unwired: 1 in, 1 out]
      n147 = shared-variable "RT CompactRIO Target\\Mod5\\PWM1"(w906) -> ()  [unwired: 1 in, 1 out]
      n148 = shared-variable "RT CompactRIO Target\\Mod5\\PWM2"(w905) -> ()  [unwired: 1 in, 1 out]
      n149 = shared-variable "RT CompactRIO Target\\Mod5\\PWM3"(w904) -> ()  [unwired: 1 in, 1 out]
    }
    frame #5 {
      n150 = local read "op-space pos\n(global frame)"() -> (w926:dbl[])
      n151 = node-c288("Loop time (ms)") -> (w925:T5)  [unwired: 3 in]
      n152 = timed-loop {
        shift-right: [w1134] -> _
        shift-left: _ -> [w1133]
        shift-right: ["Manual position control"] -> _
        shift-left: FALSE ("Manual position control") -> [w1101]
        shift-right: [w1048] -> _
        shift-left: w926 -> [w928]
        shift-right: ["Eight maze on"] -> _
        shift-left: _ -> [w1117]
        timing: w925 -> [_]
        timing-out: [_] -> w924
        shift-right: ["End Wheel"] -> _
        shift-left: _ -> [w936]
        i -> [w1092]
        stop <- "RETURN TO HOME \nPOSITION AND STOP" stop-if-true
        w933 = dbl[] [0.005, 0.005, 0.0, 0.1] ("upper limit")
        w1017 = 3 ("index (row)")
        w1018 = 1 ("index (row)")
        w1019 = 3 ("index (row)")
        w1020 = 1 ("index (row)")
        w1090 = 0 ("index (row)")
        w1091 = 0 ("index (row)")
        n153 = node-c288() -> ()  [unwired: 1 in, 1 out]
        n154 = local read "Loop seq."() -> (w943:dbl)
        n155 = local read "op-space pos\n(global frame)"() -> (w989:dbl[])
        n156 = local read "Eight maze on"() -> (w956:bool)
        n157 = Equal To 0?(x=w943) -> (x = 0?=w942:bool)
        n158 = Build Array("X", "Y", "Z", "Yaw") -> (w1054:dbl[])
        n159 = local read "Joint_pos (rad)"() -> (w1062:dbl[])
        n160 = Add(x="manual position\n(global frame)", y=w1054) -> (x+y=w957:dbl[])
        n161 = global read "Global 1.vi" "F_measured"() -> (w967:dbl[])
        n162 = Or(x="Begin Wheel", y="End Wheel") -> (x .or. y?=w951:bool)
        n163 = case shown="False" w956 {
          tunnel: [w1195 w1243] -> w958
          tunnel: w957 -> [w1196 w1244]
          tunnel: w928 -> [w1202 _]
          frame False {
            n164 = local read "Begin Wheel"() -> (w1199:bool)
            n165 = local read "End Wheel"() -> (w1198:bool)
            n166 = Index Array(array=w1202, index=1) -> (element=w1200:dbl)
            n167 = mathscript code="m = -0.004/0.290;\n\nzadjust = ypos*m;"("ypos"=w1200) -> ("zadjust"=w1193:dbl)  [unwired: 1 in, 1 out]
            n168 = Or(x=w1199, y=w1198) -> (x .or. y?=w1197:bool)
            n169 = In Range and Coerce(upper limit=0.004, x=w1193, lower limit=0.0) -> (coerced(x)=w1194:dbl)  [unwired: 1 out]
            n170 = case shown="True" w1197 {
              tunnel: w1196 -> [w1203 w1209]
              tunnel: w1194 -> [_ w1206]
              tunnel: [w1203 w1204] -> w1195
              frame False {
              }
              frame True {
                n171 = Replace Array Subset(array=dbl[] [0.0, 0.0, 0.0, 0.0] ("y"), new element=w1206, index=2) -> (w1205:dbl[])
                n172 = Add(x=w1209, y=w1205) -> (x+y=w1204:dbl[])
              }
            }
          }
          frame True {
            n173 = local read "op-space pos\n(global frame)"() -> (w1241:dbl[])
            n174 = Index Array(array=w1241, index=1) -> (element=w1247:dbl)
            n175 = In Range and Coerce(upper limit="Lego1", x=w1247, lower limit="Lego2") -> (In Range?=w1235:bool)  [unwired: 1 out]
            n176 = Index Array(array=w1241, index=0) -> (element=w1240:dbl)
            n177 = In Range and Coerce(upper limit=0.1, x=w1240, lower limit=-0.1) -> (In Range?=w1237:bool)  [unwired: 1 out]
            n178 = Not(x=w1237) -> (.not. x?=w1234:bool)
            n179 = And(x=w1234, y=w1235) -> (x .and. y?=w1236:bool)
            n180 = case shown="True" w1236 {
              tunnel: w1244 -> [w1249 w1252]
              tunnel: [w1249 w1250] -> w1243
              frame False {
              }
              frame True {
                n181 = Add(x=w1252, y=dbl[] [0.0, 0.0, 0.002, 0.0]) -> (x+y=w1250:dbl[])
              }
            }
          }
        }
        n182 = case shown="True" w942 {
          tunnel: "c" -> [w1168 w1170]
          tunnel: [w1168 w1169] -> w945
          frame False {
          }
          frame True {
            w1172 = 0 ("index (row)")
            n183 = Replace Array Subset(array=w1170, new element="cx start", index (row)=w1172, index (col)=w1172) -> (w1169:dbl[][])
          }
        }
        n184 = case shown="True" "Eight maze on" {
          tunnel: [w1174 w1182] -> w1099
          tunnel: [w1173 w1181] -> w1087
          tunnel: dbl[] [0.0, 0.0, 0.0, 0.0] ("array") -> [w1175 w1178]
          tunnel: w951 -> [w1173 _]
          frame False {
            n185 = case shown="True" w1173 {
              tunnel: w1175 -> [w1176 _]
              tunnel: [w1176 dbl[] [1.0, 1.0, 0.0, 1.0] ("array")] -> w1174
              frame False {
              }
              frame True {
              }
            }
          }
          frame True {
            n186 = Boolean To (0,1)(Boolean="Yaw_tajectory") -> (0, 1=w1189:i16)
            n187 = Boolean To (0,1)(Boolean="Y_trajectory") -> (0, 1=w1190:i16)
            n188 = Or(x="Y_trajectory", y="Yaw_tajectory") -> (x .or. y?=w1181:bool)
            n189 = To Double Precision Float(number=w1189) -> (double precision float=w1183:dbl)
            n190 = To Double Precision Float(number=w1190) -> (double precision float=w1187:dbl)
            n191 = Build Array(w1187, w1187) -> (w1186:dbl[])
            n192 = Replace Array Subset(array=w1178, new element=w1186, index=0) -> (w1184:dbl[])
            n193 = Replace Array Subset(array=w1184, new element=w1183, index=3) -> (w1182:dbl[])
          }
        }
        n194 = Index Array(array=w989, index=1) -> (element=w986:dbl)
        n195 = local read "Dzone y 2"() -> (w972:dbl)
        n196 = Index Array(array=w1062, index=0) -> (element=w1064:dbl)
        n197 = Index Array(array=w1062, index=1) -> (element=w1063:dbl)
        n198 = Index Array(array=w1062, index=2) -> (element=w1061:dbl)
        n199 = Index Array(array=w1062, index=3) -> (element=w1060:dbl)
        n200 = In Range and Coerce(upper limit=0.0 ("lower limit"), x=w986, lower limit=w972) -> (In Range?=w987:bool)  [unwired: 1 out]
        n201 = call "cRIO_4DoF_Force_conversion.vi"("Manual force"="Manual force", "F_measured"=w967, "Manual forces in"="Manual forces\n(mouse frame)") -> ("Force control"=w960:dbl[], "F_mouse"=→"Mouse forces":dbl[])  [unwired: 7 in]
        n202 = call "cRIO_4DoF_Delta_forward_kinematics.vi"("theta3"=w1061, "theta2"=w1063, "theta1"=w1064) -> ("YD"=w1067:cdb, "ZD"=w1068:cdb, "discriminant (>0)"=→"discriminant (>0)":dbl, "XD"=w1066:cdb)  [unwired: 5 in]
        n203 = case shown="True" w987 {
          tunnel: w945 -> [w1296 w1299]
          tunnel: [w1296 w1298] -> w985
          frame False {
          }
          frame True {
            w1300 = 3 ("index (row)")
            n204 = Replace Array Subset(array=w1299, new element="cTrans", index (row)=w1300, index (col)=w1300) -> (w1298:dbl[][])
          }
        }
        n205 = Greater?(x="End Wheel", y=w936) -> (0:w935:bool)
        n206 = local read "Loop_L"() -> (w971:bool)
        n207 = local read "Loop_R"() -> (w970:bool)
        n208 = Less?(x=w1092, y=10) -> (x < y?=w939:bool)
        n209 = call "cRIO_4DoF_Gonio_forward_kinematics.vi"("X in"=w1066, "Y in"=w1067, "Z in"=w1068, "Theta6_meas"=w1060) -> ("X out"=w1077:dbl, "Y out"=w1076:dbl, "Z out"=w1075:dbl, "yaw"=w1074:dbl)  [unwired: 7 in, 1 out]
        n210 = call "cRIO_4DOF_Jacobian_v3.vi"("XD"=w1066, "YD"=w1067, "ZD"=w1068, "Joint positions"=w1062) -> ("J"=w1078:dbl[][])  [unwired: 7 in]
        "J" <- w1078
        n211 = Multiply(x="deltapos", y=w1099) -> (x*y=w1097:dbl[])
        n212 = case shown="True" w935 {
          frame False {
          }
          frame True {
            n213 = local write "No LEDs"(TRUE ("No LEDs")) -> ()
          }
        }
        n214 = Or(x=w971, y=w970) -> (x .or. y?=w969:bool)
        n215 = Multiply(x=w1097, y="Trajectory scale") -> (x*y=w1086:dbl[])
        n216 = call "cRIO_4DoF_PluckerTrans.vi"("Force control"=w960, "d_{1}_{2} (mm)"="d_{1}_{2} (mm)") -> ("TransF"=w962:dbl[])  [unwired: 9 in]
        "TransF" <- w962
        n217 = case shown="True" w969 {
          tunnel: "m" -> [w1256 w1279]
          tunnel: [w1256 w1278] -> w1001
          tunnel: [w1255 w1277] -> w1000
          tunnel: w985 -> [w1255 w1276]
          frame False {
          }
          frame True {
            n218 = local read "op-space pos\n(global frame)"() -> (w1270:dbl[])
            n219 = Index Array(array=w1270, index=1) -> (element=w1272:dbl)
            n220 = Index Array(array="MDzone", index=0) -> (element=w1274:dbl)
            n221 = Index Array(array="MDzone", index=1) -> (element=w1269:dbl)
            n222 = local read "Loop_L"() -> (w1267:bool)
            n223 = local read "BB1_L"() -> (w1260:bool)
            n224 = local read "Loop_R"() -> (w1266:bool)
            n225 = In Range and Coerce(upper limit=w1274, x=w1272, lower limit=w1269) -> (In Range?=w1262:bool)  [unwired: 1 out]
            n226 = local read "BB1_R"() -> (w1257:bool)
            n227 = Not(x=w1260) -> (.not. x?=w1259:bool)
            n228 = Not(x=w1257) -> (.not. x?=w1258:bool)
            n229 = And(x=w1267, y=w1259) -> (x .and. y?=w1265:bool)
            n230 = And(x=w1266, y=w1258) -> (x .and. y?=w1264:bool)
            n231 = Or(x=w1265, y=w1264) -> (x .or. y?=w1263:bool)
            n232 = And(x=w1263, y=w1262) -> (x .and. y?=w1261:bool)
            n233 = case shown="True" w1261 {
              tunnel: w1279 -> [w1287 w1293]
              tunnel: [w1286 w1292] -> w1278
              tunnel: [w1285 w1290] -> w1277
              tunnel: w1276 -> [w1280 w1291]
              frame False {
                w1283 = 0 ("index (row)")
                w1284 = 0 ("index (row)")
                n234 = Replace Array Subset(array=w1287, new element="mLoop", index (row)=w1284, index (col)=w1284) -> (w1286:dbl[][])
                n235 = Replace Array Subset(array=w1280, new element="cLoop", index (row)=w1283, index (col)=w1283) -> (w1285:dbl[][])
              }
              frame True {
                w1294 = 0 ("index (row)")
                w1295 = 0 ("index (row)")
                n236 = Replace Array Subset(array=w1293, new element="mMD", index (row)=w1295, index (col)=w1295) -> (w1292:dbl[][])
                n237 = Replace Array Subset(array=w1291, new element="cMD", index (row)=w1294, index (col)=w1294) -> (w1290:dbl[][])
              }
            }
          }
        }
        "m_applied" <- w1001
        "c_applied" <- w1000
        n238 = Array To Cluster(array=w1086) -> (cluster=→"Trajectory changes in XY":T4)
        n239 = Build Array(w1077, w1076, w1075, w1074) -> (w931:dbl[])
        n240 = Array To Cluster(array=w1086) -> (cluster=→"Trajectory changes in Yaw":T4)
        n241 = Negate(x="delpos limits (+/-) \ntrajectory control\n(global frame)") -> (-x=w1106:dbl[])
        n242 = Negate(x=w933) -> (-x=w932:dbl[])
        n243 = In Range and Coerce(upper limit="delpos limits (+/-) \ntrajectory control\n(global frame)", x=w1086, lower limit=w1106) -> (coerced(x)=w1088:dbl[])  [unwired: 1 out]
        n244 = call "cRIO_4DoF_Encoders_countsvel2radvel(subVI).vi"() -> ("Joint_space_velocity"=w1040:dbl[])  [unwired: 11 in]
        "velocity \n(joint space)" <- w1040
        n245 = In Range and Coerce(upper limit=w933, x="Global offset", lower limit=w932) -> (coerced(x)=w930:dbl[])  [unwired: 1 out]
        n246 = mathscript code="Joint_vel = Joint_vel';\n\nOp_vel = J*Joint_vel;\n\nOp_vel = real(Op_vel);"("J"=w1078, "Joint_vel"=w1040) -> ("Op_vel"=w1096:dbl[][])  [unwired: 1 in, 1 out]
        n247 = case shown="True" "Ftrans" {
          tunnel: w962 -> [_ w1254]
          tunnel: [w1253 w1254] -> w961
          tunnel: w960 -> [w1253 _]
          frame False {
          }
          frame True {
          }
        }
        n248 = case shown="True" w1087 {
          tunnel: [dbl[] [0.0, 0.0, 0.0, 0.0] w1320] -> w1089
          tunnel: w1088 -> [_ w1320]
          frame False {
          }
          frame True {
          }
        }
        "changes from trajectory" <- w1089
        n249 = Greater?(x="Eight maze on", y=w1117) -> (0:w1115:bool)
        n250 = Less?(x="Eight maze on", y=w1117) -> (x < y?=w1116:bool)
        n251 = Or(x=w1115, y=w1116) -> (x .or. y?=→"Eightmaze_switch":bool)
        n252 = Add(x=w931, y=w930) -> (x+y=w929:dbl[])
        "op-space pos\n(global frame)" <- w929
        n253 = Or(x="Manual position control", y=w939) -> (x .or. y?=w941:bool)
        n254 = call "cRIO_4DoF_Fsense_deadband(subVI).vi"("Fsense deadband (Nm or N)"="Fsense deadband\n (Nm or N)", "Enable Fsense Deadband"=TRUE, "F_{2} in"=w961) -> ("F_{2} out"=w1071:dbl[])  [unwired: 8 in]
        n255 = Reshape Array(w1096, 4 ("dimension size")) -> (w1073:dbl[])
        "velocity\n(global frame)" <- w1073
        n256 = call "cRIO_4DoF_InvYaw_global2mouse_v2.vi"("op-space pos"=w929, "op_vel"=w1073) -> ("vel_out"=w1044:dbl[])  [unwired: 9 in]
        "velocity \n(mouseframe)" <- w1044
        n257 = Negate(x="Mouse force limits") -> (-x=w1110:dbl[])
        n258 = In Range and Coerce(upper limit="Mouse force limits", x=w1071, lower limit=w1110) -> (coerced(x)=w1046:dbl[])  [unwired: 1 out]
        n259 = local read "Loop time (ms)"() -> (w1045:i64)
        n260 = call "cRIO_4DoF_Admittance_controller_v3.vi"("F"=w1046, "v_2 in"=w1044, "c"=w1000, "m"=w1001, "Loop time (ms)"=w1045) -> ("del_m"=w1047:dbl[])  [unwired: 9 in, 1 out]
        n261 = local read "op-space pos\n(global frame)"() -> (w1083:dbl[])
        n262 = local read "Yaw_tajectory"() -> (w1082:bool)
        n263 = local read "deltapos"() -> (w1084:dbl[])
        n264 = call "cRIO_4DoF_deactivate_mouseforce_axes.vi"("Disable Yaw forces"="Disable Yaw forces", "Disable X"="Disable X", "Disable Y forces"="Disable Y forces", "Disable -X"="Disable -X", "del_m in"=w1047) -> ("del_m out"=w1081:dbl[])  [unwired: 6 in]
        n265 = disable-structure shown="Enabled" {
          disable-tunnel: w1084 -> [w1311 _]
          disable-tunnel: w1083 -> [w1310 w1316]
          disable-tunnel: w1082 -> [w1309 _]
          disable-tunnel: [w1308 w1316] -> w1043
          frame Disabled {
            n266 = case shown="True" w1309 {
              tunnel: w1311 -> [_ w1315]
              tunnel: w1310 -> [w1312 w1314]
              tunnel: [w1312 w1313] -> w1308
              frame False {
              }
              frame True {
                n267 = Add(x=w1315, y=w1314) -> (x+y=w1313:dbl[])
              }
            }
          }
          frame Enabled {
          }
        }
        n268 = local read "op-space pos\n(global frame)"() -> (w1125:dbl[])
        n269 = Multiply(x=w1081, y="Admittance scale") -> (x*y=w1079:dbl[])
        n270 = Index Array(array=w1043, index=3) -> (element=w1041:dbl)
        n271 = Negate(x="delpos limits (+/-)\nadmittance control \n(mouse frame)") -> (-x=w1108:dbl[])
        n272 = In Range and Coerce(upper limit="delpos limits (+/-)\nadmittance control \n(mouse frame)", x=w1079, lower limit=w1108) -> (coerced(x)=w1022:dbl[])  [unwired: 1 out]
        "changes from \nadmittance {m}" <- w1022
        n273 = local read "J"() -> (w1122:dbl[][])
        n274 = call "cRIO_4DoF_Yaw_mouse2global_v2.vi"("yawangle"=w1041, "Mouse forces"=w1022) -> ("F_2"=w999:dbl[])  [unwired: 9 in]
        n275 = local read "Begin Wheel"() -> (w952:bool)
        n276 = local read "End Wheel"() -> (w949:bool)
        n277 = local read "Radius"() -> (w993:dbl)
        n278 = local read "Loop_L"() -> (w991:bool)
        n279 = local read "Loop_R"() -> (w990:bool)
        n280 = local read "op-space pos\n(global frame)"() -> (w992:dbl[])
        n281 = local read "Dzone"() -> (w997:bool)
        n282 = Not(x=w997) -> (.not. x?=w996:bool)
        n283 = Not(x=w952) -> (.not. x?=w953:bool)
        n284 = Not(x=w949) -> (.not. x?=w948:bool)
        n285 = Compound Arithmetic op=AND("Vector correction", w996, w953, w948) -> (w994:bool)
        n286 = case shown="False" w994 {
          tunnel: w999 -> [w1301 w1304]
          tunnel: [w1301 w1302] -> w998
          tunnel: w993 -> [_ w1303]
          tunnel: w992 -> [_ w1305]
          tunnel: w991 -> [_ w1307]
          tunnel: w990 -> [_ w1306]
          frame False {
          }
          frame True {
            n287 = call "cRIO_4DoF_vectorcompensation_eightplus.vi"("F_2"=w1304, "Radius"=w1303, "op-space pos\n(global frame)"=w1305, "Loop_R"=w1306, "Loop_L"=w1307) -> ("delPosout"=w1302:dbl[])  [unwired: 6 in]
          }
        }
        n288 = Compound Arithmetic op=ADD(w928, w998, w1089) -> (w1121:dbl[])
        n289 = case shown="False" w941 {
          tunnel: w1121 -> [w1389 _]
          tunnel: [w1388 w1400] -> w1049
          tunnel: w958 -> [w1390 w1401]
          tunnel: w939 -> [_ w1396]
          tunnel: w1101 -> [_ w1395]
          tunnel: "Manual position control" -> [_ w1394]
          frame False {
            w1392 = 2 ("index")
            n290 = Array Subset(array=w1390, index=w1392, length=1) -> (w1393:dbl[])
            n291 = Replace Array Subset(array=w1389, new element=w1393, index=w1392) -> (w1388:dbl[])
          }
          frame True {
            n292 = local read "Eightmaze_switch"() -> (w1397:bool)
            n293 = Greater?(x=w1394, y=w1395) -> (0:w1398:bool)
            n294 = Compound Arithmetic op=OR(w1396, w1398, w1397) -> (w1399:bool)
            n295 = case shown="False" w1399 {
              tunnel: [w1402 w1404] -> w1400
              tunnel: w1401 -> [w1402 _]
              frame False {
              }
              frame True {
                w1403 = 0.0 ("Z")
                n296 = local read "op-space pos\n(global frame)"() -> (w1404:dbl[])
                n297 = local write "manual position\n(global frame)"(w1404) -> ()
                n298 = local write "target position"(w1404) -> ()
                n299 = local write "Yaw"(w1403) -> ()
                n300 = local write "X"(w1403) -> ()
                n301 = local write "Y"(w1403) -> ()
                n302 = local write "Z"(w1403) -> ()
              }
            }
          }
        }
        n303 = In Range and Coerce(upper limit="upper limit", x=w1049, lower limit="lower limit") -> (coerced(x)=w1048:dbl[])  [unwired: 1 out]
        "target position" <- w1048
        n304 = call-poly <vilib>:"PID.vi"("output range"="Output range (PWM)", "PID gains"="Admittance PID gains", "process variable"=w1125, "setpoint"=w1048) -> ("output"=w1023:dbl[])  [unwired: 6 in, 1 out]
        n305 = mathscript code="opspace = [op_vel]';\njointspace = inv(J)*opspace;\nlinrad = real(jointspace(1:3,1));\nrotrad = real(jointspace(4,1));" "Velocity conversion (in PWM space)"("op_vel"=w1023, "J"=w1122) -> ("linrad"=w1136:dbl[], "rotrad"=w1139:dbl)  [unwired: 1 in, 1 out]
        n306 = Compound Arithmetic op=OR(w939, "Disable PID", "Out of range") -> (w1130:bool)
        n307 = local read "c_applied"() -> (w1015:dbl[][])
        n308 = local read "m_applied"() -> (w1016:dbl[][])
        n309 = Add(x=w1136, y="delta PWM offset") -> (x+y=w1138:dbl[])
        n310 = Tick Count (ms)() -> (millisecond timer value=w938:u32)
        n311 = Add(x=w1139, y="goniometer PWM\n offset") -> (x+y=w1137:dbl)
        n312 = case shown="False" w1130 {
          tunnel: w1138 -> [w1499 _]
          tunnel: w1137 -> [w1498 _]
          tunnel: [w1499 w1500] -> w1126
          tunnel: [w1498 w1501] -> w1024
          tunnel: "goniometer PWM\n offset" -> [_ w1501]
          tunnel: "delta PWM offset" -> [_ w1500]
          frame False {
          }
          frame True {
          }
        }
        n313 = Index Array(array=w1015, index (row)=w1091, index (col)=w1091) -> (element=w1014:dbl)
        n314 = Index Array(array=w1016, index (row)=w1090, index (col)=w1090) -> (element=w1011:dbl)
        n315 = local read "SynPulseOn"() -> (w947:bool)
        n316 = local read "MD_L"() -> (w984:bool)
        n317 = local read "MD_R"() -> (w983:bool)
        n318 = local read "Sound"() -> (w982:bool)
        n319 = local read "AIR"() -> (w981:bool)
        n320 = To Double Precision Float(number=w938) -> (double precision float=w1104:dbl)
        n321 = Index Array(array=w1016, index (row)=w1018, index (col)=w1018) -> (element=w1010:dbl)
        n322 = Index Array(array=w1015, index (row)=w1020, index (col)=w1020) -> (element=w1013:dbl)
        n323 = local read "op-space pos\n(global frame)"() -> (w1162:dbl[])
        n324 = local read "changes from \nadmittance {m}"() -> (w1161:dbl[])
        n325 = Index Array(array=w1016, index (row)=w1017, index (col)=w1017) -> (element=w1009:dbl)
        n326 = Index Array(array=w1015, index (row)=w1019, index (col)=w1019) -> (element=w1012:dbl)
        n327 = Or(x=w984, y=w983) -> (x .or. y?=w980:bool)
        n328 = local read "Mouse forces"() -> (w1114:dbl[])
        n329 = local read "Joint_pos (rad)"() -> (w1163:dbl[])
        n330 = Build Array(w1014, w1013, w1012) -> (w1008:dbl[])
        n331 = Build Array(w1011, w1010, w1009) -> (w1007:dbl[])
        n332 = Build Array(w982, w981, w980, w947) -> (w979:bool[])
        n333 = Boolean To (0,1)(Boolean=w979) -> (0, 1=w978:i16[])
        n334 = To Double Precision Float(number=w978) -> (double precision float=w977:dbl[])
        n335 = Build Array (concatenate)(w1163, w1162, w1161, w1104, w1126, w1024, w1114, w1008, w1007, w977) -> (w1160:dbl[])
        n336 = Index Array(array=w1126, index=1) -> (element=w1026:dbl)
        n337 = Index Array(array=w1126, index=2) -> (element=w1025:dbl)
        n338 = Index Array(array=w1126, index=0) -> (element=w1027:dbl)
        n339 = Decimate 1D Array(w1160) -> (w1159:dbl[], w1158:dbl[], w1157:dbl[], w1156:dbl[], w1155:dbl[], w1154:dbl[], w1153:dbl[], w1152:dbl[], w1151:dbl[], w1150:dbl[], w1149:dbl[], w1148:dbl[], w1147:dbl[], w1146:dbl[], w1145:dbl[], w1144:dbl[], w1143:dbl[], w1142:dbl[], w1141:dbl[], w1053:dbl[], w1052:dbl[], w1051:dbl[], w1050:dbl[], w1006:dbl[], w1005:dbl[], w1004:dbl[], w1003:dbl[], w976:dbl[], w975:dbl[], w974:dbl[], w946:dbl[])
        n340 = In Range and Coerce(upper limit=99.0, x=w1027, lower limit=1.0) -> (coerced(x)=w1031:dbl)  [unwired: 1 out]
        n341 = In Range and Coerce(upper limit=99.0, x=w1026, lower limit=1.0) -> (coerced(x)=w1030:dbl)  [unwired: 1 out]
        n342 = In Range and Coerce(upper limit=99.0, x=w1025, lower limit=1.0) -> (coerced(x)=w1029:dbl)  [unwired: 1 out]
        n343 = In Range and Coerce(upper limit=99.0, x=w1024, lower limit=1.0) -> (coerced(x)=w1028:dbl)  [unwired: 1 out]
        n344 = Build Array(w1159, w1158, w1157, w1156, w1155, w1154, w1153, w1152, w1151, w1150, w1149, w1148, w1147, w1146, w1145, w1144, w1143, w1142, w1141, w1053, w1052, w1051, w1050, w1006, w1005, w1004, w1003, w976, w975, w974, w946) -> (→"Data output":dbl[][])
        n345 = Tick Count (ms)() -> (millisecond timer value=w1134:u32)
        n346 = shared-variable "RT CompactRIO Target\\Mod5\\PWM2"(w1029) -> ()  [unwired: 1 in, 1 out]
        n347 = shared-variable "RT CompactRIO Target\\Mod5\\PWM0"(w1031) -> ()  [unwired: 1 in, 1 out]
        n348 = Subtract(x=w1134, y=w1133) -> (x-y=→"True loop time (ms)":u32)
        n349 = shared-variable "RT CompactRIO Target\\Mod5\\PWM1"(w1030) -> ()  [unwired: 1 in, 1 out]
        n350 = shared-variable "RT CompactRIO Target\\Mod5\\PWM3"(w1028) -> ()  [unwired: 1 in, 1 out]
        n351 = disable-structure shown="Enabled" {
          disable-tunnel: w1126 -> [w1322 _]
          disable-tunnel: w1024 -> [w1321 _]
          frame Enabled {
            n352 = local read "changes from \nadmittance {m}"() -> (w1324:dbl[])
            n353 = local read "Mouse forces"() -> (w1323:dbl[])
            n354 = local read "op-space pos\n(global frame)"() -> (w1346:dbl[])
            n355 = Array Subset(array=w1324, index=0, length=3) -> (w1332:dbl[])
            n356 = Array Subset(array=w1324, index=3, length=1) -> (w1327:dbl[])
            n357 = Build Array (concatenate)(w1322, w1321) -> (w1344:dbl[])
            n358 = Array Subset(array=w1323, index=0, length=3) -> (w1340:dbl[])
            n359 = Array Subset(array=w1323, index=3, length=1) -> (w1335:dbl[])
            n360 = Array To Cluster(array=w1346) -> (cluster=→"XY position" →"Z position" →"alpha beta gamma":T8)
            n361 = Array To Cluster(array=w1327) -> (cluster=→"Admittance changes in Yaw":T4)
            n362 = Array To Cluster(array=w1332) -> (cluster=→"Admittance changes in XY":T4)
            n363 = Reshape Array(w1344, 4 ("dimension size")) -> (w1342:dbl[])
            n364 = Array To Cluster(array=w1335) -> (cluster=→"Torques (Nm)":T4)
            n365 = Array To Cluster(array=w1340) -> (cluster=→"Forces (N)":T4)
            n366 = Array To Cluster(array=w1342) -> (cluster=→"PWM":T4)
          }
          frame Disabled {
          }
        }
        n367 = node-c288() -> ()  [unwired: 1 in, 1 out]
        "loop" <- w1092
        "Eight maze on" <- "Eight maze on"
      }
      n368 = node-c288(w924) -> ()  [unwired: 1 out]
    }
    frame #6 {
      n369 = while "Joint space control" {
        stop <- FALSE stop-if-true
        n370 = local read "Joint_pos (rad)"() -> (w1523:dbl[])
        n371 = local read "theta1,2,3"() -> (w1528:dbl)
        n372 = local read "theta6"() -> (w1527:dbl)
        n373 = Build Array(w1528, w1528, w1528, w1527) -> (w1536:dbl[])
        n374 = local read "Theta output range"() -> (w1524:cluster{"output high":dbl, "output low":dbl}[])
        n375 = local read "Theta PID gains"() -> (w1525:T2)
        n376 = call-poly <vilib>:"PID.vi"("output range"=w1524, "PID gains"=w1525, "process variable"=w1523, "setpoint"=w1536) -> ("output"=w1531:dbl[])  [unwired: 6 in, 1 out]
        n377 = Add(x=w1531, y=dbl[] [50.0, 50.0, 50.0, 50.0]) -> (x+y=w1529:dbl[])
        n378 = Index Array(array=w1529, index=0) -> (element=w1510:dbl)
        n379 = Index Array(array=w1529, index=1) -> (element=w1509:dbl)
        n380 = Index Array(array=w1529, index=2) -> (element=w1508:dbl)
        n381 = Index Array(array=w1529, index=3) -> (element=w1507:dbl)
        n382 = In Range and Coerce(upper limit=99.0, x=w1510, lower limit=1.0) -> (coerced(x)=w1514:dbl)  [unwired: 1 out]
        n383 = In Range and Coerce(upper limit=99.0, x=w1509, lower limit=1.0) -> (coerced(x)=w1513:dbl)  [unwired: 1 out]
        n384 = In Range and Coerce(upper limit=99.0, x=w1508, lower limit=1.0) -> (coerced(x)=w1512:dbl)  [unwired: 1 out]
        n385 = In Range and Coerce(upper limit=99.0, x=w1507, lower limit=1.0) -> (coerced(x)=w1511:dbl)  [unwired: 1 out]
        n386 = shared-variable "RT CompactRIO Target\\Mod5\\PWM0"(w1514) -> ()  [unwired: 1 in, 1 out]
        n387 = shared-variable "RT CompactRIO Target\\Mod5\\PWM2"(w1512) -> ()  [unwired: 1 in, 1 out]
        n388 = shared-variable "RT CompactRIO Target\\Mod5\\PWM1"(w1513) -> ()  [unwired: 1 in, 1 out]
        n389 = shared-variable "RT CompactRIO Target\\Mod5\\PWM3"(w1511) -> ()  [unwired: 1 in, 1 out]
      }
      n390 = local write "Record to current file"(FALSE ("Record to current file")) -> ()
    }
  }
  n391 = flat-sequence {
    frame #0 {
      w1538 = FALSE
      w1541 = bool[] [TRUE, FALSE, TRUE, FALSE, TRUE, FALSE, TRUE, FALSE, TRUE, FALSE, TRUE, FALSE, TRUE, FALSE, TRUE, FALSE, TRUE, FALSE, TRUE, FALSE, TRUE, FALSE, TRUE, FALSE, TRUE, FALSE, TRUE, FALSE, TRUE, FALSE, TRUE, FALSE, TRUE, FALSE, TRUE, FALSE, TRUE, FALSE, TRUE, FALSE, TRUE, FALSE, TRUE, FALSE, TRUE, FALSE, TRUE, FALSE, TRUE, FALSE, TRUE, FALSE, TRUE, FALSE, TRUE, FALSE, TRUE, FALSE, TRUE, FALSE, TRUE, FALSE, TRUE, FALSE, TRUE, FALSE, TRUE, FALSE, TRUE, FALSE, TRUE]  # Alternating
      (unwired) bool[] [TRUE, FALSE, FALSE, TRUE, FALSE, TRUE, TRUE, FALSE, TRUE, FALSE, FALSE, TRUE, FALSE, TRUE, FALSE, FALSE, TRUE, FALSE, TRUE, TRUE, FALSE, TRUE, FALSE, FALSE, TRUE, FALSE, TRUE, TRUE, FALSE, TRUE, FALSE, FALSE, TRUE, FALSE, TRUE, TRUE, FALSE, TRUE, FALSE, FALSE, TRUE, FALSE, TRUE, TRUE, FALSE, TRUE, FALSE, FALSE, TRUE, FALSE, TRUE, TRUE, FALSE, TRUE, FALSE, FALSE, TRUE, FALSE, TRUE, TRUE, FALSE, TRUE, FALSE, FALSE, TRUE, FALSE, TRUE, TRUE, FALSE, TRUE, FALSE]  # Psuedo random
      w1537 = TRUE
      w1540 = FALSE
      n392 = local write "All BBR"(w1538) -> ()
      n393 = local write "All BBL"(w1538) -> ()
      n394 = local write "BB3_R"(w1538) -> ()
      n395 = local write "BB1_R"(w1538) -> ()
      n396 = local write "BB3_L"(w1538) -> ()
      n397 = local write "BB1_L"(w1538) -> ()
      n398 = local write "BB2_R"(w1538) -> ()
      n399 = local write "BB2_L"(w1538) -> ()
      n400 = local write "Initialize"(w1537) -> ()
      n401 = local write "Servo enable"(w1537) -> ()
      n402 = local write "Sound"(w1537) -> ()
      n403 = local write "No Milk"(w1540) -> ()
      n404 = shared-variable "RT CompactRIO Target\\Mod6\\DIO29"(w1540) -> ()  [unwired: 1 in, 1 out]
      n405 = shared-variable "RT CompactRIO Target\\Mod6\\DIO14"(w1540) -> ()  [unwired: 1 in, 1 out]
      n406 = shared-variable "RT CompactRIO Target\\Mod6\\DIO20"(w1540) -> ()  [unwired: 1 in, 1 out]
      n407 = shared-variable "RT CompactRIO Target\\Mod6\\DIO30"(w1540) -> ()  [unwired: 1 in, 1 out]
      n408 = shared-variable "RT CompactRIO Target\\Mod6\\DIO7"(w1540) -> ()  [unwired: 1 in, 1 out]
      n409 = shared-variable "RT CompactRIO Target\\Mod6\\DIO20"(w1540) -> ()  [unwired: 1 in, 1 out]
      n410 = shared-variable "RT CompactRIO Target\\Mod6\\DIO17"(w1537) -> ()  [unwired: 1 in, 1 out]
      n411 = local write "Loop seq."(0.0 ("Loop seq.")) -> ()
      n412 = local write "MDsetup"(FALSE ("MDsetup")) -> ()
      n413 = local write "PWM positions"(dbl[] [9.5, 8.1, 5.1, 5.8]) -> ()
      "Direction array" <- w1541
    }
    frame #1 {
      n414 = while "Loop sequence Right" {
        stop <- FALSE stop-if-true
        n415 = flat-sequence {
          frame #0 {
            # "Check sequence for right turn"
            n416 = while {
              stop <- w1631 stop-if-true
              n417 = local read "Right"() -> (w1631:bool)
              n418 = Wait (ms)(milliseconds to wait=u32 10) -> ()  [unwired: 1 out]
            }
          }
          frame #1 {
            # "Breakbeam 1 Left"
            n419 = while {
              shift-right: [w1634] -> _
              shift-left: FALSE -> [w1638]
              stop <- w1633 stop-if-true
              n420 = shared-variable "RT CompactRIO Target\\Mod6\\DIO15"() -> (w1634:bool)  [unwired: 1 in, 1 out]
              n421 = Wait (ms)(milliseconds to wait=u32 10) -> ()  [unwired: 1 out]
              n422 = local read "Initialize"() -> (w1635:bool)
              n423 = Less?(x=w1634, y=w1638) -> (x < y?=w1636:bool)
              n424 = Or(x=w1636, y=w1635) -> (x .or. y?=w1633:bool)
              "BB1_L" <- w1633
            }
          }
          frame #2 {
            # "Breakbeam 2 Right"
            n425 = while {
              stop <- w1640 stop-if-true
              w1640 = TRUE ("BB2_R")
              n426 = Wait (ms)(milliseconds to wait=u32 10) -> ()  [unwired: 1 out]
              "BB2_R" <- w1640
            }
            n427 = local write "Initialize"(FALSE ("Initialize")) -> ()
          }
          frame #3 {
            # "Breakbeam 3 Right"
            n428 = while {
              shift-right: [w1643] -> _
              shift-left: _ -> [w1645]
              stop <- w1642 stop-if-true
              n429 = shared-variable "RT CompactRIO Target\\Mod6\\DIO13"() -> (w1643:bool)  [unwired: 1 in, 1 out]
              n430 = Wait (ms)(milliseconds to wait=u32 10) -> ()  [unwired: 1 out]
              n431 = Less?(x=w1643, y=w1645) -> (x < y?=w1642:bool)
              "BB3_R" <- w1642
            }
          }
          frame #4 {
            n432 = local write "Servo enable"(TRUE) -> ()
            n433 = Wait (ms)(milliseconds to wait=u32 50) -> ()  [unwired: 1 out]
          }
          frame #5 {
            # "Servo 1 position"
            n434 = local read "PWM positions"() -> (w1651:dbl[])
            n435 = Wait (ms)(milliseconds to wait=u32 50) -> ()  [unwired: 1 out]
            n436 = Replace Array Subset(array=w1651, new element=9.5 ("new element/subarray"), index=0) -> (w1648:dbl[])
            n437 = local write "PWM positions"(w1648) -> ()
            "All BBR" <- TRUE
          }
          frame #6 {
            # "Wait for mouse to reach MD stop point"
            n438 = while {
              shift-right: [w1656] -> _
              shift-left: _ -> [w1659]
              stop <- w1658 stop-if-true
              n439 = local read "op-space pos\n(global frame)"() -> (w1660:dbl[])
              n440 = Wait (ms)(milliseconds to wait=u32 10) -> ()  [unwired: 1 out]
              n441 = local read "MDstopR"() -> (w1655:dbl)
              n442 = Index Array(array=w1660, index=1) -> (element=w1656:dbl)
              n443 = Less?(x=w1656, y=w1655) -> (x < y?=w1662:bool)
              n444 = Greater?(x=w1659, y=w1655) -> (0:w1661:bool)
              n445 = And(x=w1662, y=w1661) -> (x .and. y?=w1658:bool)
            }
          }
          frame #7 {
            w1665 = FALSE
            # "Disable X and reset indicators"
            n446 = local write "Disable X"(TRUE ("Disable X")) -> ()
            n447 = local write "All BBR"(w1665) -> ()
            n448 = local write "BB1_R"(w1665) -> ()
            n449 = local write "BB1_L"(w1665) -> ()
            n450 = local write "BB2_R"(w1665) -> ()
            n451 = local write "BB3_R"(w1665) -> ()
            n452 = Wait (ms)(milliseconds to wait=u32 10) -> ()  [unwired: 1 out]
          }
          frame #8 {
            n453 = local write "MDsetup"(TRUE ("MDsetup")) -> ()
            n454 = Wait (ms)(milliseconds to wait=u32 50) -> ()  [unwired: 1 out]
          }
          frame #9 {
            # "Move to position"
            n455 = while {
              stop <- w1675 stop-if-true
              n456 = local read "op-space pos\n(global frame)"() -> (w1669:dbl[])
              n457 = local read "MDsRy"() -> (w1668:dbl)
              n458 = local read "MDstopR"() -> (w1676:dbl)
              n459 = Array Subset(array=w1669, index=0, length=2) -> (w1672:dbl[])
              n460 = Build Array(w1668, w1676) -> (w1680:dbl[])
              n461 = local read "MDpos_lims"() -> (w1674:dbl[])
              n462 = Subtract(x=w1680, y=w1672) -> (x-y=w1679:dbl[])
              n463 = Negate(x=w1674) -> (-x=w1678:dbl[])
              n464 = In Range and Coerce(upper limit=w1674, x=w1679, lower limit=w1678) -> (In Range?=w1677:bool[])  [unwired: 1 out]
              n465 = And Array Elements(Boolean array=w1677) -> (logical AND=w1675:bool)
              n466 = Wait (ms)(milliseconds to wait=u32 10) -> ()  [unwired: 1 out]
            }
          }
          frame #10 {
            # "Raise MD servo"
            n467 = local read "PWM positions"() -> (w1682:dbl[])
            n468 = local read "PWMset2"() -> (w1683:dbl[])
            n469 = Wait (ms)(milliseconds to wait=u32 10) -> ()  [unwired: 1 out]
            n470 = Index Array(array=w1683, index=1) -> (element=w1684:dbl)
            n471 = Replace Array Subset(array=w1682, new element=w1684, index=2) -> (w1681:dbl[])
            n472 = local write "PWM positions"(w1681) -> ()
          }
          frame #11 {
            # "Milk dispense"
            n473 = local write "MD_R"(TRUE ("MD_R")) -> ()
            n474 = Wait (ms)(milliseconds to wait=u32 100) -> ()  [unwired: 1 out]
          }
          frame #12 {
            # "Pause"
            n475 = local read "MD time (ms)"() -> (w1690:i32)
            n476 = Add(x=w1690, y=u32 1000 ("milliseconds to wait")) -> (x+y=w1692:u32)
            n477 = Wait (ms)(milliseconds to wait=w1692) -> ()  [unwired: 1 out]
          }
          frame #13 {
            # "Lower MD servo"
            n478 = local read "PWMset1"() -> (w1699:dbl[])
            n479 = local read "PWM positions"() -> (w1698:dbl[])
            n480 = Index Array(array=w1699, index=1) -> (element=w1696:dbl)
            n481 = Replace Array Subset(array=w1698, new element=w1696, index=2) -> (w1697:dbl[])
            n482 = local write "PWM positions"(w1697) -> ()
            n483 = Wait (ms)(milliseconds to wait=u32 100) -> ()  [unwired: 1 out]
          }
          frame #14 {
            # "Play a beep sound"
            n484 = flat-sequence {
              frame #0 {
                n485 = local write "Sound"(FALSE ("Sound")) -> ()
                n486 = Wait (ms)(milliseconds to wait=u32 250) -> ()  [unwired: 1 out]
              }
              frame #1 {
                n487 = local write "Sound"(TRUE ("Sound")) -> ()
                n488 = Wait (ms)(milliseconds to wait=u32 500) -> ()  [unwired: 1 out]
              }
            }
          }
          frame #15 {
            # "Enable X"
            n489 = local write "MDsetup"(FALSE ("MDsetup")) -> ()
            n490 = Wait (ms)(milliseconds to wait=u32 100) -> ()  [unwired: 1 out]
            n491 = local write "Disable X"(FALSE ("Disable X")) -> ()
          }
        }
      }
      n492 = while "Loop sequence Left" {
        stop <- FALSE stop-if-true
        n493 = flat-sequence {
          frame #0 {
            # "Check sequence for left turn"
            n494 = while {
              stop <- w1730 stop-if-true
              n495 = local read "Left"() -> (w1730:bool)
              n496 = Wait (ms)(milliseconds to wait=u32 10) -> ()  [unwired: 1 out]
            }
          }
          frame #1 {
            # "Breakbeam 1 Right"
            n497 = while {
              shift-right: [w1732] -> _
              shift-left: FALSE -> [w1737]
              stop <- w1733 stop-if-true
              n498 = shared-variable "RT CompactRIO Target\\Mod6\\DIO31"() -> (w1732:bool)  [unwired: 1 in, 1 out]
              n499 = Wait (ms)(milliseconds to wait=u32 10) -> ()  [unwired: 1 out]
              n500 = local read "Initialize"() -> (w1734:bool)
              n501 = Less?(x=w1732, y=w1737) -> (x < y?=w1735:bool)
              n502 = Or(x=w1735, y=w1734) -> (x .or. y?=w1733:bool)
              "BB1_R" <- w1733
            }
          }
          frame #2 {
            # "Breakbeam 2 Left"
            n503 = while {
              stop <- w1739 stop-if-true
              w1739 = TRUE ("BB2_L")
              n504 = Wait (ms)(milliseconds to wait=u32 10) -> ()  [unwired: 1 out]
              "BB2_L" <- w1739
            }
            n505 = local write "Initialize"(FALSE ("Initialize")) -> ()
          }
          frame #3 {
            # "Breakbeam 3 Left"
            n506 = while {
              shift-right: [w1742] -> _
              shift-left: _ -> [w1744]
              stop <- w1741 stop-if-true
              n507 = shared-variable "RT CompactRIO Target\\Mod6\\DIO21"() -> (w1742:bool)  [unwired: 1 in, 1 out]
              n508 = Wait (ms)(milliseconds to wait=u32 10) -> ()  [unwired: 1 out]
              n509 = Less?(x=w1742, y=w1744) -> (x < y?=w1741:bool)
              "BB3_L" <- w1741
            }
          }
          frame #4 {
            n510 = local write "Servo enable"(TRUE) -> ()
            n511 = Wait (ms)(milliseconds to wait=u32 50) -> ()  [unwired: 1 out]
          }
          frame #5 {
            # "Servo 1 position"
            n512 = local read "PWM positions"() -> (w1750:dbl[])
            n513 = Wait (ms)(milliseconds to wait=u32 50) -> ()  [unwired: 1 out]
            n514 = Replace Array Subset(array=w1750, new element=4.5 ("new element/subarray"), index=0) -> (w1747:dbl[])
            n515 = local write "PWM positions"(w1747) -> ()
            "All BBL" <- TRUE
          }
          frame #6 {
            # "Wait for mouse to reach MD stop point"
            n516 = while {
              shift-right: [w1759] -> _
              shift-left: _ -> [w1758]
              stop <- w1755 stop-if-true
              n517 = local read "op-space pos\n(global frame)"() -> (w1761:dbl[])
              n518 = Wait (ms)(milliseconds to wait=u32 10) -> ()  [unwired: 1 out]
              n519 = local read "MDstopL"() -> (w1753:dbl)
              n520 = Index Array(array=w1761, index=1) -> (element=w1759:dbl)
              n521 = Less?(x=w1759, y=w1753) -> (x < y?=w1757:bool)
              n522 = Greater?(x=w1758, y=w1753) -> (0:w1756:bool)
              n523 = And(x=w1757, y=w1756) -> (x .and. y?=w1755:bool)
            }
          }
          frame #7 {
            w1762 = FALSE
            # "Disable X and reset indicators"
            n524 = Wait (ms)(milliseconds to wait=u32 10) -> ()  [unwired: 1 out]
            n525 = local write "Disable X"(TRUE ("Disable X")) -> ()
            n526 = local write "All BBL"(w1762) -> ()
            n527 = local write "BB1_L"(w1762) -> ()
            n528 = local write "BB1_R"(w1762) -> ()
            n529 = local write "BB2_L"(w1762) -> ()
            n530 = local write "BB3_L"(w1762) -> ()
          }
          frame #8 {
            n531 = local write "MDsetup"(TRUE ("MDsetup")) -> ()
            n532 = Wait (ms)(milliseconds to wait=u32 50) -> ()  [unwired: 1 out]
          }
          frame #9 {
            # "Move to position"
            n533 = while {
              stop <- w1773 stop-if-true
              n534 = local read "MDstopL"() -> (w1779:dbl)
              n535 = local read "op-space pos\n(global frame)"() -> (w1768:dbl[])
              n536 = local read "MDsLy"() -> (w1767:dbl)
              n537 = local read "MDpos_lims"() -> (w1776:dbl[])
              n538 = Build Array(w1767, w1779) -> (w1778:dbl[])
              n539 = Array Subset(array=w1768, index=0, length=2) -> (w1769:dbl[])
              n540 = Subtract(x=w1778, y=w1769) -> (x-y=w1777:dbl[])
              n541 = Negate(x=w1776) -> (-x=w1775:dbl[])
              n542 = In Range and Coerce(upper limit=w1776, x=w1777, lower limit=w1775) -> (In Range?=w1774:bool[])  [unwired: 1 out]
              n543 = And Array Elements(Boolean array=w1774) -> (logical AND=w1773:bool)
              n544 = Wait (ms)(milliseconds to wait=u32 10) -> ()  [unwired: 1 out]
            }
          }
          frame #10 {
            # "Raise MD servo"
            n545 = local read "PWM positions"() -> (w1783:dbl[])
            n546 = local read "PWMset1"() -> (w1780:dbl[])
            n547 = Index Array(array=w1780, index=2) -> (element=w1781:dbl)
            n548 = Wait (ms)(milliseconds to wait=u32 10) -> ()  [unwired: 1 out]
            n549 = Replace Array Subset(array=w1783, new element=w1781, index=3) -> (w1785:dbl[])
            n550 = local write "PWM positions"(w1785) -> ()
          }
          frame #11 {
            # "Milk dispense"
            n551 = local write "MD_L"(TRUE ("MD_L")) -> ()
            n552 = Wait (ms)(milliseconds to wait=u32 100) -> ()  [unwired: 1 out]
          }
          frame #12 {
            # "Pause"
            n553 = local read "MD time (ms)"() -> (w1790:i32)
            n554 = Add(x=w1790, y=u32 1000 ("milliseconds to wait")) -> (x+y=w1789:u32)
            n555 = Wait (ms)(milliseconds to wait=w1789) -> ()  [unwired: 1 out]
          }
          frame #13 {
            # "Lower MD servo"
            n556 = local read "PWM positions"() -> (w1796:dbl[])
            n557 = local read "PWMset2"() -> (w1798:dbl[])
            n558 = Index Array(array=w1798, index=2) -> (element=w1795:dbl)
            n559 = Wait (ms)(milliseconds to wait=u32 100) -> ()  [unwired: 1 out]
            n560 = Replace Array Subset(array=w1796, new element=w1795, index=3) -> (w1797:dbl[])
            n561 = local write "PWM positions"(w1797) -> ()
          }
          frame #14 {
            # "Play a beep sound"
            n562 = flat-sequence {
              frame #0 {
                n563 = local write "Sound"(FALSE ("Sound")) -> ()
                n564 = Wait (ms)(milliseconds to wait=u32 250) -> ()  [unwired: 1 out]
              }
              frame #1 {
                n565 = local write "Sound"(TRUE ("Sound")) -> ()
                n566 = Wait (ms)(milliseconds to wait=u32 500) -> ()  [unwired: 1 out]
              }
            }
          }
          frame #15 {
            # "Enable X"
            n567 = local write "MDsetup"(FALSE ("MDsetup")) -> ()
            n568 = local write "Disable X"(FALSE ("Disable X")) -> ()
            n569 = Wait (ms)(milliseconds to wait=u32 100) -> ()  [unwired: 1 out]
          }
        }
      }
      n570 = while "Control outputs, Inputs, and Left/Right switch" {
        stop <- FALSE stop-if-true
        w1837 = dbl[] [9.5, 8.1, 5.1, 5.8]
        n571 = shared-variable "RT CompactRIO Target\\Mod6\\DIO15"() -> (w1833:bool)  [unwired: 1 in, 1 out]
        n572 = shared-variable "RT CompactRIO Target\\Mod6\\DIO31"() -> (w1827:bool)  [unwired: 1 in, 1 out]
        n573 = shared-variable "RT CompactRIO Target\\Mod6\\DIO21"() -> (w1828:bool)  [unwired: 1 in, 1 out]
        n574 = shared-variable "RT CompactRIO Target\\Mod6\\DIO28"() -> (w1830:bool)  [unwired: 1 in, 1 out]
        n575 = shared-variable "RT CompactRIO Target\\Mod6\\DIO13"() -> (w1831:bool)  [unwired: 1 in, 1 out]
        n576 = shared-variable "RT CompactRIO Target\\Mod6\\DIO5"() -> (w1829:bool)  [unwired: 1 in, 1 out]
        n577 = feedback #1(w1837) -> (w1838:dbl[])
        n578 = feedback #2(w1837) -> (w1841:dbl[])
        n579 = Build Array(w1833, w1827, w1828, w1829, w1830, w1831) -> (→"appended array":bool[])
        n580 = In Range and Coerce(upper limit=w1841, x="PWM positions", lower limit=w1838) -> (coerced(x)=w1840:dbl[])  [unwired: 1 out]
        n581 = Subtract(x=w1840, y="PWM rate") -> (x-y=w1839:dbl[])
        n582 = Add(x=w1840, y="PWM rate") -> (x+y=w1842:dbl[])
        n583 = feedback-in #1(w1839) -> ()
        n584 = feedback-in #2(w1842) -> ()
        n585 = Index Array(array=w1840, index=0) -> (element=w1824:dbl)
        n586 = Index Array(array=w1840, index=1) -> (element=w1823:dbl)
        n587 = Index Array(array=w1840, index=2) -> (element=w1850:dbl)
        n588 = Index Array(array=w1840, index=3) -> (element=w1851:dbl)
        n589 = local read "Direction array"() -> (w1821:bool[])
        n590 = shared-variable "RT CompactRIO Target\\Mod5\\PWM7"(w1824) -> ()  [unwired: 1 in, 1 out]
        n591 = shared-variable "RT CompactRIO Target\\Mod5\\PWM4"(w1823) -> ()  [unwired: 1 in, 1 out]
        n592 = shared-variable "RT CompactRIO Target\\Mod5\\PWM5"(w1850) -> ()  [unwired: 1 in, 1 out]
        n593 = shared-variable "RT CompactRIO Target\\Mod5\\PWM6"(w1851) -> ()  [unwired: 1 in, 1 out]
        n594 = Index Array(array=w1821, index="Loop seq.") -> (element=w1822:bool)
        "Left" <- w1822
        n595 = case shown="False" "No LED no Sound" {
          tunnel: "LED_L" -> [w1862 _]
          tunnel: "LED_R" -> [w1861 _]
          tunnel: "Sound" -> [w1860 _]
          tunnel: [w1862 FALSE ("LED_L")] -> w1813
          tunnel: [w1861 FALSE ("LED_R")] -> w1812
          tunnel: [w1860 TRUE ("Sound")] -> w1816
          frame False {
          }
          frame True {
          }
        }
        n596 = Not(x=w1822) -> (.not. x?=→"Right":bool)
        n597 = case shown="True" "Flash LEDs" {
          tunnel: w1813 -> [w1857 _]
          tunnel: [w1857 "LED_L 2"] -> w1811
          tunnel: w1812 -> [w1856 _]
          tunnel: [w1856 "LED_R 2"] -> w1809
          frame False {
          }
          frame True {
          }
        }
        n598 = case shown="True" "No LEDs" {
          tunnel: w1811 -> [w1853 _]
          tunnel: [w1853 FALSE ("LED_L 2")] -> w1810
          tunnel: w1809 -> [w1852 _]
          tunnel: [w1852 FALSE ("LED_R 2")] -> w1808
          frame False {
          }
          frame True {
          }
        }
        n599 = shared-variable "RT CompactRIO Target\\Mod6\\DIO18"("Servo enable") -> ()  [unwired: 1 in, 1 out]
        n600 = shared-variable "RT CompactRIO Target\\Mod6\\DIO17"(w1816) -> ()  [unwired: 1 in, 1 out]
        n601 = shared-variable "RT CompactRIO Target\\Mod6\\DIO29"("MD_L") -> ()  [unwired: 1 in, 1 out]
        n602 = shared-variable "RT CompactRIO Target\\Mod6\\DIO14"("MD_R") -> ()  [unwired: 1 in, 1 out]
        n603 = shared-variable "RT CompactRIO Target\\Mod6\\DIO6"("AIR") -> ()  [unwired: 1 in, 1 out]
        n604 = shared-variable "RT CompactRIO Target\\Mod6\\DIO20"(w1810) -> ()  [unwired: 1 in, 1 out]
        n605 = shared-variable "RT CompactRIO Target\\Mod6\\DIO30"(w1808) -> ()  [unwired: 1 in, 1 out]
        n606 = Wait (ms)(milliseconds to wait=u32 5) -> ()  [unwired: 1 out]
      }
      n607 = while {
        i -> [w1612]
        stop <- FALSE stop-if-true
        n608 = flat-sequence {
          frame #0 {
            n609 = while {
              stop <- w1615 stop-if-true
              n610 = local read "All BBR"() -> (w1616:bool)
              n611 = local read "All BBL"() -> (w1617:bool)
              n612 = Or(x=w1617, y=w1616) -> (x .or. y?=w1615:bool)
              n613 = Wait (ms)(milliseconds to wait=u32 50) -> ()  [unwired: 1 out]
            }
          }
          frame #1 {
            n614 = for {
              N: 1 -> [_]
              n615 = local read "Loop seq."() -> (w1622:dbl)
              n616 = Add(x=w1622, y=1.0) -> (x+y=w1620:dbl)
              n617 = local write "Loop seq."(w1620) -> ()
            }
          }
          frame #2 {
            n618 = while {
              stop <- w1623 stop-if-true
              n619 = local read "All BBR"() -> (w1626:bool)
              n620 = local read "All BBL"() -> (w1627:bool)
              n621 = Not(x=w1626) -> (.not. x?=w1624:bool)
              n622 = Not(x=w1627) -> (.not. x?=w1625:bool)
              n623 = Wait (ms)(milliseconds to wait=u32 50) -> ()  [unwired: 1 out]
              n624 = And(x=w1625, y=w1624) -> (x .and. y?=w1623:bool)
            }
          }
        }
        n625 = Wait (ms)(milliseconds to wait=u32 100) -> ()  [unwired: 1 out]
        "Seq update" <- w1612
      }
      n626 = while "Sound timing" {
        shift-right: [w1596] -> _
        shift-left: FALSE ("BB1_L") -> [w1595]
        shift-right: [w1590] -> _
        shift-left: FALSE ("BB1_R") -> [w1591]
        stop <- FALSE stop-if-true
        n627 = local read "BB1_L"() -> (w1590:bool)
        n628 = local read "BB1_R"() -> (w1596:bool)
        n629 = Wait (ms)(milliseconds to wait=u32 50) -> ()  [unwired: 1 out]
        n630 = Greater?(x=w1596, y=w1595) -> (0:w1589:bool)
        n631 = Greater?(x=w1590, y=w1591) -> (0:w1588:bool)
        n632 = local read "Left"() -> (w1594:bool)
        n633 = Compound Arithmetic op=OR(w1588, w1589, "Repeat sound") -> (w1587:bool)
        n634 = And(x=w1587, y=w1594) -> (x .and. y?=w1593:bool)
        n635 = case shown="False" w1593 {
          tunnel: w1587 -> [w1600 _]
          frame False {
            n636 = local read "Right"() -> (w1599:bool)
            n637 = And(x=w1600, y=w1599) -> (x .and. y?=w1598:bool)
            n638 = case shown="True" w1598 {
              frame False {
              }
              frame True {
                n639 = for {
                  N: 4 -> [_]
                  n640 = flat-sequence {
                    frame #0 {
                      n641 = local write "Sound"(FALSE ("Sound")) -> ()
                      n642 = Wait (ms)(milliseconds to wait=u32 250) -> ()  [unwired: 1 out]
                    }
                    frame #1 {
                      n643 = local write "Repeat sound"(FALSE ("Repeat sound")) -> ()
                      n644 = local write "Sound"(TRUE ("Sound")) -> ()
                      n645 = Wait (ms)(milliseconds to wait=u32 500) -> ()  [unwired: 1 out]
                    }
                  }
                }
              }
            }
          }
          frame True {
            n646 = flat-sequence {
              frame #0 {
                n647 = local write "Sound"(FALSE ("Sound")) -> ()
                n648 = Wait (ms)(milliseconds to wait=u32 3000) -> ()  [unwired: 1 out]
              }
              frame #1 {
                n649 = local write "Sound"(TRUE ("Sound")) -> ()
                n650 = Wait (ms)(milliseconds to wait=u32 50) -> ()  [unwired: 1 out]
              }
              frame #2 {
                n651 = local write "Repeat sound"(FALSE ("Repeat sound")) -> ()
              }
            }
          }
        }
      }
      n652 = while {
        stop <- FALSE stop-if-true
        n653 = flat-sequence {
          frame #0 {
            n654 = while {
              stop <- w1581 stop-if-true
              n655 = local read "AIR"() -> (w1581:bool)
              n656 = Wait (ms)(milliseconds to wait=u32 50) -> ()  [unwired: 1 out]
            }
          }
          frame #1 {
            n657 = Wait (ms)(milliseconds to wait="Air puff time") -> ()  [unwired: 1 out]
          }
          frame #2 {
            n658 = Wait (ms)(milliseconds to wait=u32 50) -> ()  [unwired: 1 out]
            n659 = local write "AIR"(FALSE ("AIR_L")) -> ()
          }
        }
        n660 = Wait (ms)(milliseconds to wait=u32 50) -> ()  [unwired: 1 out]
      }
      n661 = while {
        stop <- FALSE stop-if-true
        n662 = flat-sequence {
          frame #0 {
            n663 = while {
              stop <- w1549 stop-if-true
              n664 = local read "Servo enable"() -> (w1549:bool)
              n665 = Wait (ms)(milliseconds to wait=u32 50) -> ()  [unwired: 1 out]
            }
          }
          frame #1 {
            n666 = Wait (ms)(milliseconds to wait="servo wait (ms)") -> ()  [unwired: 1 out]
          }
          frame #2 {
            n667 = local write "Servo enable"(FALSE ("Servo enable")) -> ()
          }
        }
        n668 = Wait (ms)(milliseconds to wait=u32 50) -> ()  [unwired: 1 out]
      }
      n669 = while "Servo 2 position and LEDs" {
        stop <- FALSE stop-if-true
        n670 = local read "PWM positions"() -> (w1709:dbl[])
        n671 = local read "Left"() -> (w1710:bool)
        n672 = Wait (ms)(milliseconds to wait=u32 50) -> ()  [unwired: 1 out]
        n673 = case shown="True" w1710 {
          tunnel: w1709 -> [w1718 w1726]
          tunnel: [w1717 w1725] -> w1708
          frame False {
            n674 = local read "PWMset1"() -> (w1714:dbl[])
            n675 = local write "LED_L"(FALSE ("LED_L")) -> ()
            n676 = local write "LED_R"(TRUE ("LED_R")) -> ()
            n677 = Index Array(array=w1714, index=0) -> (element=w1713:dbl)
            n678 = Replace Array Subset(array=w1718, new element=w1713, index=1) -> (w1717:dbl[])
          }
          frame True {
            n679 = local read "PWMset2"() -> (w1722:dbl[])
            n680 = local write "LED_R"(FALSE ("LED_R")) -> ()
            n681 = local write "LED_L"(TRUE ("LED_L")) -> ()
            n682 = Index Array(array=w1722, index=0) -> (element=w1720:dbl)
            n683 = Replace Array Subset(array=w1726, new element=w1720, index=1) -> (w1725:dbl[])
          }
        }
        n684 = local write "PWM positions"(w1708) -> ()
      }
      n685 = while {
        stop <- FALSE stop-if-true
        n686 = flat-sequence {
          frame #0 {
            n687 = while {
              stop <- w1565 stop-if-true
              n688 = local read "MD_R"() -> (w1565:bool)
              n689 = Wait (ms)(milliseconds to wait=u32 50) -> ()  [unwired: 1 out]
            }
          }
          frame #1 {
            n690 = local read "No Milk"() -> (w1566:bool)
            n691 = case shown="False" w1566 {
              frame False {
                n692 = local read "MD time (ms)"() -> (w1567:i32)
                n693 = Wait (ms)(milliseconds to wait=w1567) -> ()  [unwired: 1 out]
              }
              frame True {
                n694 = Wait (ms)(milliseconds to wait=u32 50) -> ()  [unwired: 1 out]
              }
            }
          }
          frame #2 {
            w1569 = FALSE ("MD_R")
            n695 = Wait (ms)(milliseconds to wait=u32 50) -> ()  [unwired: 1 out]
            n696 = local write "MD_R"(w1569) -> ()
            n697 = local write "No Milk"(w1569) -> ()
          }
        }
      }
      n698 = while {
        stop <- FALSE stop-if-true
        n699 = flat-sequence {
          frame #0 {
            n700 = while {
              stop <- w1573 stop-if-true
              n701 = local read "MD_L"() -> (w1573:bool)
              n702 = Wait (ms)(milliseconds to wait=u32 50) -> ()  [unwired: 1 out]
            }
          }
          frame #1 {
            n703 = local read "No Milk"() -> (w1574:bool)
            n704 = case shown="False" w1574 {
              frame False {
                n705 = local read "MD time (ms)"() -> (w1575:i32)
                n706 = Wait (ms)(milliseconds to wait=w1575) -> ()  [unwired: 1 out]
              }
              frame True {
                n707 = Wait (ms)(milliseconds to wait=u32 50) -> ()  [unwired: 1 out]
              }
            }
          }
          frame #2 {
            w1577 = FALSE ("MD_L")
            n708 = Wait (ms)(milliseconds to wait=u32 50) -> ()  [unwired: 1 out]
            n709 = local write "MD_L"(w1577) -> ()
            n710 = local write "No Milk"(w1577) -> ()
          }
        }
      }
      n711 = while {
        stop <- FALSE stop-if-true
        n712 = flat-sequence {
          frame #0 {
            n713 = while {
              stop <- w1553 stop-if-true
              n714 = local read "Flash LEDs"() -> (w1553:bool)
              n715 = Wait (ms)(milliseconds to wait=u32 250) -> ()  [unwired: 1 out]
            }
          }
          frame #1 {
            n716 = for {
              N: 10 -> [_]
              n717 = flat-sequence {
                frame #0 {
                  n718 = local write "LED_L 2"(TRUE ("LED_L")) -> ()
                  n719 = local write "LED_R 2"(TRUE ("LED_R")) -> ()
                  n720 = Wait (ms)(milliseconds to wait=u32 1000) -> ()  [unwired: 1 out]
                }
                frame #1 {
                  n721 = local write "LED_R 2"(FALSE ("LED_R")) -> ()
                  n722 = local write "LED_L 2"(FALSE ("LED_L")) -> ()
                  n723 = Wait (ms)(milliseconds to wait=u32 1000) -> ()  [unwired: 1 out]
                }
              }
            }
          }
          frame #2 {
            n724 = local write "Flash LEDs"(FALSE ("Mouse off")) -> ()
          }
        }
      }
    }
  }
  n725 = node-c288(i64 1 ("Period")) -> (w3:T5)  [unwired: 3 in]
  n726 = while "Avoid Delta robot joint collision with platform" {
    stop <- FALSE stop-if-true
    n727 = local read "Joint_pos (rad)"() -> (w1872:dbl[])
    n728 = Wait (ms)(milliseconds to wait=u32 25) -> ()  [unwired: 1 out]
    n729 = Array Subset(array=w1872, index=0, length=3) -> (w1869:dbl[])
    n730 = Less?(x=w1869, y=dbl[] [-0.85, -0.85, -0.85]) -> (x < y?=w1874:bool[])
    n731 = Or Array Elements(Boolean array=w1874) -> (logical OR=w1866:bool)
    n732 = local write "Out of range"(w1866) -> ()
  }
  n733 = while "Encoder counts to Joint position" {
    stop <- FALSE stop-if-true
    n734 = local read "Loop time (ms)"() -> (w1887:i64)
    n735 = call "cRIO_4DoF_Encoders_counts2rad(subVI).vi"() -> ("Theta3"=w1882:dbl, "Theta2"=w1883:dbl, "Theta1"=w1884:dbl, "Theta6"=w1888:dbl)  [unwired: 4 in]
    n736 = Build Array(w1884, w1883, w1882, w1888) -> (w1881:dbl[])
    n737 = Divide "offset"(x=3.141592653589793, y=4.0) -> (x/y=w1880:dbl)
    n738 = Wait (ms)(milliseconds to wait=w1887) -> ()  [unwired: 1 out]
    n739 = Build Array(w1880, w1880, w1880, 0.0 ("element")) -> (w1878:dbl[])
    n740 = Subtract(x=w1881, y=w1878) -> (x-y=w1877:dbl[])
    n741 = Subtract(x=w1877, y="Joint offset") -> (x-y=→"Joint_pos (rad)":dbl[])
  }
  n742 = timed-loop {
    timing: w3 -> [_]
    timing-out: [_] -> w2
    stop <- FALSE stop-if-true
    n743 = node-c288() -> ()  [unwired: 1 in, 1 out]
    n744 = local read "Sensor V offset"() -> (w1893:dbl[])
    n745 = call "cRIO_4DoF_Fsample.vi"("Sensor V offset"=w1893) -> ("F"=→"F":dbl[], "Array"=→"Raw voltages":dbl[])  [unwired: 9 in]
    n746 = node-c288() -> ()  [unwired: 1 in, 1 out]
  }
  n747 = node-c288(w2) -> ()  [unwired: 1 out]
  n748 = while "Force sensor voltages to Forces and torques" {
    stop <- FALSE stop-if-true
    n749 = local read "Loop time (ms)"() -> (w1901:i64)
    n750 = Wait (ms)(milliseconds to wait=w1901) -> ()  [unwired: 1 out]
    n751 = flat-sequence {
      tunnel: [w1910] -> w1898
      tunnel: "number Fsamples" -> [w1909]
      tunnel: w1898 -> [w1916]
      tunnel: [w1915] -> w1897
      frame #0 {
        n752 = for {
          N: w1909 -> [_]
          tunnel: [w1913] -> w1911 mode=indexing
          n753 = Wait (ms)(milliseconds to wait=u32 1) -> ()  [unwired: 1 out]
          n754 = local read "F"() -> (w1913:dbl[])
        }
        n755 = Transpose 2D Array(2D array=w1911) -> (transposed array=w1910:dbl[][])
      }
      frame #1 {
        n756 = for {
          N: 4 -> [_]
          tunnel: w1916 -> [w1918] mode=indexing
          tunnel: [w1917] -> w1915 mode=indexing
          n757 = call-poly <vilib>:"Mean.vi"("X"=w1918) -> ("mean"=w1917:dbl)  [unwired: 1 out]
        }
      }
    }
    n758 = Array Subset(array=w1897, index=0, length=3) -> (w1900:dbl[])
    n759 = Array Subset(array=w1897, index=3, length=1) -> (w1899:dbl[])
    n760 = global write "Global 1.vi" "F_measured"(w1897) -> ()
    n761 = Array To Cluster(array=w1900) -> (cluster=→"Forces (N) 2":T4)
    n762 = Array To Cluster(array=w1899) -> (cluster=→"Torques (Nm) 2":T4)
    "F_measured" <- w1897
  }
  n763 = while "Data saving loop... a new file needs to be created for each data set using the \"Write data to file (PC VI).vi\"" {
    stop <- FALSE stop-if-true
    n764 = flat-sequence "Data Saving" {
      tunnel: [w1933] -> w1926
      tunnel: [w1934] -> w1925
      tunnel: w1926 -> [w1936]
      tunnel: [w1936] -> w1922
      tunnel: w1925 -> [w1935]
      tunnel: [w1935] -> w1920
      tunnel: w1922 -> [w1941]
      tunnel: [w1941] -> w1921
      tunnel: w1920 -> [w1940]
      tunnel: [w1940] -> w1919
      tunnel: w1921 -> [w1943]
      tunnel: w1919 -> [w1944]
      tunnel: [w1942] -> w1924
      tunnel: w1924 -> [w1961]
      frame #0 {
        # "Open network stream endpoint"
        n765 = local write "Data syncing"(FALSE ("Activate")) -> ()
        n766 = Create Network Stream Writer Endpoint(7:1000 ("writer buffer size"), 9:dbl[][] [] ("appended array"), 11:"cRIO_Write_Data" ("writer name")) -> (0:w1931:errorcluster, 3:w1932:refnum<k21>)  [unwired: 4 in]
        n767 = Flush Stream(8:w1931, 11:w1932) -> (0:w1933:errorcluster, 3:w1934:refnum<k21>)  [unwired: 2 in, 1 out]
      }
      frame #1 {
        # "Begin Saving Data"
        n768 = while {
          stop <- "BEGIN saving new data set" stop-if-true
          n769 = Wait (ms)(milliseconds to wait=u32 250) -> ()  [unwired: 1 out]
        }
      }
      frame #2 {
        # "Start Pulse Sync loop"
        n770 = local write "Data syncing"(TRUE) -> ()
      }
      frame #3 {
        # "Save Data by writing elements to network stream -/-/-/-/ and Pause Saving if necessary, by increasing loop time"
        n771 = while {
          tunnel: w1944 -> [w1951]
          tunnel: w1943 -> [w1950]
          tunnel: [w1946] -> w1942
          stop <- "STOP saving data set" stop-if-true
          n772 = local read "Data output"() -> (w1945:dbl[][])
          n773 = shared-variable-write "Write Single Element to Stream"(w1951, w1950, w1945) -> (w1954:refnum<k21>, →"network stream":errorcluster)  [unwired: 1 in, 1 out]
          n774 = property class="Network Stream Endpoint"(reference=w1954) -> (reference out=w1946:refnum<k21>, "AvailElmntsForWrite"=→"Available Elements for Writing in network stream":i32)  [unwired: 1 in, 1 out]
          n775 = case shown="False" "PAUSE saving data set" {
            tunnel: [w1955 "PAUSE ms to wait"] -> w1947
            frame False {
              n776 = local read "Loop time (ms)"() -> (w1955:i64)
            }
            frame True {
            }
          }
          n777 = Wait (ms)(milliseconds to wait=w1947) -> ()  [unwired: 1 out]
        }
      }
      frame #4 {
        # "Stop"
        n778 = Flush Stream(11:w1961) -> (3:w1962:refnum<k21>)  [unwired: 3 in, 2 out]
        n779 = local write "BEGIN saving new data set"(FALSE ("BEGIN SAVING DATA")) -> ()
        n780 = local write "Data syncing"(FALSE ("Data syncing")) -> ()
        n781 = local write "STOP saving data set"(FALSE ("STOP SAVING DATA")) -> ()
        n782 = local write "PAUSE saving data set"(FALSE ("PAUSE SAVING DATA")) -> ()
        n783 = Destroy Stream Endpoint(11:w1962) -> ()  [unwired: 1 in, 1 out]
      }
    }
  }
  n784 = while {
    stop <- FALSE stop-if-true
    n785 = local read "op-space pos\n(global frame)"() -> (w1980:dbl[])
    n786 = local read "Dzone y 2"() -> (w1964:dbl)
    n787 = local read "Dzone x"() -> (w1968:dbl)
    n788 = Index Array(array=w1980, index=1) -> (element=w1965:dbl)
    n789 = Index Array(array=w1980, index=0) -> (element=w1969:dbl)
    n790 = Add(x=w1968, y=0.001) -> (x+y=w1966:dbl)
    n791 = Negate(x=w1966) -> (-x=w1979:dbl)
    n792 = In Range and Coerce(upper limit=w1966, x=w1969, lower limit=w1979) -> (In Range?=w1978:bool)  [unwired: 1 out]
    n793 = Greater?(x=w1965, y=w1964) -> (0:w1963:bool)
    n794 = And(x=w1963, y=w1978) -> (x .and. y?=w1970:bool)
    "Dzone" <- w1970
    n795 = local read "Loop time (ms)"() -> (w1982:i64)
    n796 = Greater?(x=w1969, y=0.0) -> (0:w1976:bool)
    n797 = Wait (ms)(milliseconds to wait=w1982) -> ()  [unwired: 1 out]
    n798 = Not(x=w1970) -> (.not. x?=w1971:bool)
    n799 = And(x=w1976, y=w1971) -> (x .and. y?=→"Loop_R":bool)
    n800 = Less?(x=w1969, y=0.0) -> (x < y?=w1973:bool)
    n801 = And(x=w1973, y=w1971) -> (x .and. y?=→"Loop_L":bool)
  }
  n802 = while "Measure force sensor voltage offset" {
    shift-right: [w1993] -> _
    shift-left: _ -> [w1992]
    i -> [w1989]
    stop <- FALSE stop-if-true
    n803 = Wait (ms)(milliseconds to wait=u32 250) -> ()  [unwired: 1 out]
    n804 = Less?(x=w1989, y=2) -> (x < y?=w1987:bool)
    n805 = Or(x="Measure Fsensor \nV offset", y=w1987) -> (x .or. y?=w1986:bool)
    n806 = case shown="True" w1986 {
      tunnel: [w1994 w1996] -> w1993
      tunnel: w1992 -> [w1994 _]
      frame False {
      }
      frame True {
        n807 = flat-sequence {
          tunnel: [w1998] -> w1997
          tunnel: w1997 -> [w2004]
          tunnel: [w2003] -> w1995
          tunnel: [w2009] -> w1996
          tunnel: w1995 -> [w2009]
          frame #0 {
            n808 = for {
              N: 20 -> [_]
              tunnel: [w2002] -> w1999 mode=indexing
              n809 = local read "Raw voltages"() -> (w2002:dbl[])
              n810 = Wait (ms)(milliseconds to wait=u32 1) -> ()  [unwired: 1 out]
            }
            n811 = Transpose 2D Array(2D array=w1999) -> (transposed array=w1998:dbl[][])
          }
          frame #1 {
            n812 = for {
              N: 6 -> [_]
              tunnel: w2004 -> [w2007] mode=indexing
              tunnel: [w2006] -> w2003 mode=indexing
              n813 = call-poly <vilib>:"Mean.vi"("X"=w2007) -> ("mean"=w2006:dbl)  [unwired: 1 out]
            }
          }
          frame #2 {
            n814 = local write "Measure Fsensor \nV offset"(FALSE ("DAQ V offset")) -> ()
          }
        }
      }
    }
    "Sensor V offset" <- w1993
  }
  n815 = while {
    stop <- FALSE stop-if-true
    n816 = flat-sequence {
      frame #0 {
        n817 = while {
          stop <- w2011 stop-if-true
          n818 = local read "Eight maze on"() -> (w2011:bool)
          n819 = Wait (ms)(milliseconds to wait=u32 100) -> ()  [unwired: 1 out]
          n820 = case shown="False" w2011 {
            frame False {
              w2013 = FALSE
              n821 = local write "Y_trajectory"(w2013) -> ()
              n822 = local write "Yaw_tajectory"(w2013) -> ()
            }
            frame True {
            }
          }
        }
      }
      frame #1 {
        n823 = local read "op-space pos\n(global frame)"() -> (w2016:dbl[])
        n824 = Index Array(array=w2016, index=3) -> (element=w2014:dbl)
        n825 = while {
          tunnel: w2014 -> [w2037]
          stop <- w2044 stop-if-true
          n826 = local read "Half Dzone Limit"() -> (w2019:bool)
          n827 = local read "upper limit"() -> (w2031:dbl[])
          n828 = local read "op-space pos\n(global frame)"() -> (w2040:dbl[])
          n829 = local read "lower limit"() -> (w2030:dbl[])
          n830 = local read "Radius"() -> (w2027:dbl)
          n831 = local read "Gradient R"() -> (w2039:dbl)
          n832 = local read "Right"() -> (w2017:bool)
          n833 = local read "Left"() -> (w2018:bool)
          n834 = local write "delpos limits (+/-)\nadmittance control \n(mouse frame)"("delpos limits (+/-)\nadmittance control \nDzone") -> ()
          n835 = local read "Rsmall"() -> (w2023:dbl)
          n836 = local read "Dzone y"() -> (w2025:dbl)
          n837 = local read "Dzone x"() -> (w2026:dbl)
          n838 = local read "C"() -> (w2024:dbl)
          n839 = mathscript code="xpos = Pos(1,1);\nypos = Pos(1,2);\nyawpos = Pos(1,4);\n\nyaw_in = real(round((yaw_init - pi/2)/(pi))*pi + pi/2);\n\nuplim(1) = -(m*(ypos)+C+0.002);\nlowlim(1)  = -uplim(1);\n\nif ypos <0 \n    uplim(4) = yaw_in + pi/8;\n    lowlim(4) = yaw_in - pi/8;\nelse\n    yawgrad = (pi/4 - pi/8)/0.05*ypos + pi/8;\n    if yawgrad > pi/4\n        yawgrad = pi/4\n    end\n    uplim(4) = yaw_in + yawgrad;\n    lowlim(4) = yaw_in - yawgrad;\nend\n\nuplim(2) = Dy +0.0005;  % y limit = Y edge of Dzone \n\n% If Half Dzone limit button is high, then limit the \n% x and yaw range of motion to avoid mouse clash\n% with door\nif all(HDLim)\n    if all(Left)\n        uplim(1)  = 0;\n        lowlim(4) = yaw_in;\n    end\n    if all(Right)\n        lowlim(1) = 0;\n        uplim(4) = yaw_in;\n    end\nend"("Pos"=w2040, "m"=w2039, "yaw_init"=w2037, "uplim"=w2031, "lowlim"=w2030, "R"=w2027, "Dx"=w2026, "Dy"=w2025, "C"=w2024, "Rsmall"=w2023, "HDLim"=w2019, "Left"=w2018, "Right"=w2017) -> ("uplim"=w2029:dbl[], "lowlim"=w2028:dbl[])  [unwired: 1 in, 1 out]
          n840 = local read "Loop_R"() -> (w2042:bool)
          n841 = local read "Loop_L"() -> (w2043:bool)
          n842 = local read "Dzone"() -> (w2047:bool)
          n843 = local read "Eight maze on"() -> (w2046:bool)
          n844 = local write "Disable -X"("Disable -X Dzone") -> ()
          n845 = local write "Y_trajectory"(FALSE ("Mousetrack_Y")) -> ()
          n846 = local write "Disable Y forces"(FALSE ("Disable Y forces")) -> ()
          n847 = local write "Disable Yaw forces"(FALSE ("Disable Yaw forces")) -> ()
          n848 = local write "MDsetup"(FALSE ("MDsetup")) -> ()
          n849 = local write "Yaw_tajectory"(FALSE ("Mousetrack_Yaw")) -> ()
          n850 = Or(x=w2043, y=w2042) -> (x .or. y?=w2041:bool)
          n851 = local write "upper limit"(w2029) -> ()
          n852 = local write "lower limit"(w2028) -> ()
          n853 = Not(x=w2047) -> (.not. x?=w2049:bool)
          n854 = local read "Loop time (ms)"() -> (w2036:i64)
          n855 = local write "deltapos"(dbl[] [0.0, 0.0, 0.0, 0.0] ("deltapos")) -> ()
          n856 = Not(x=w2046) -> (.not. x?=w2045:bool)
          n857 = And(x=w2049, y=w2041) -> (x .and. y?=w2048:bool)
          n858 = Or(x=w2048, y=w2045) -> (x .or. y?=w2044:bool)
          n859 = Wait (ms)(milliseconds to wait=w2036) -> ()  [unwired: 1 out]
        }
      }
      frame #2 {
        n860 = while {
          stop <- w2591 stop-if-true
          n861 = local read "op-space pos\n(global frame)"() -> (w2586:dbl[])
          n862 = local read "Gradient R"() -> (w2587:dbl)
          n863 = local read "MDsetup"() -> (w2567:bool)
          n864 = local read "MDstopR"() -> (w2566:dbl)
          n865 = local read "MDstopL"() -> (w2565:dbl)
          n866 = local read "Radius"() -> (w2584:dbl)
          n867 = mathscript code="Rcen = R;     % center of right loop = (R,0)\nLcen = -R;     % center of right loop = (-R,0)\nxpos = Pos(1,1);\nypos = Pos(1,2);\nzpos = Pos(1,3);\nyawpos = Pos(1,4);\n\nRotz = [cos(yawpos),-sin(yawpos),0; sin(yawpos),cos(yawpos),0; 0,0,1];\nxhat = [1, 0, 0]';\nzhat = [0, 0, 1]';\n\nif xpos > 0    % right loop\n       xcen = xpos - Rcen;\n       ycen = ypos;\n       Rmag = real((xcen^2 + ycen^2)^0.5);\n       xtarg = R/Rmag*xcen  + Rcen;\n       ytarg = R/Rmag*ycen;      \n       RLsgn = 1;\nelse % left loop\n       xcen = xpos - Lcen;\n       ycen = ypos;\n       Rmag = real((xcen^2 + ycen^2)^0.5);\n       xtarg = R/Rmag*xcen + Lcen;\n       ytarg = R/Rmag*ycen; \n       RLsgn = -1;    \nend\n\nvecpos = [xcen, ycen, 0]';         % position vector, zero'd circle\nvecyaw = RLsgn*cross(vecpos,zhat);  % yaw vector\nvecyaw_o = Rotz'*vecyaw;        %  yaw vector transformed by actual yaw\nyawerrsign = sign(0 - vecyaw_o(2));  % sign of yaw error\nyawerrmag = acos(dot(vecyaw_o,xhat)/(norm(vecyaw_o)*norm(xhat))); % magnitude of yaw error   \nyawtarg  = yawpos - yawerrsign*real(yawerrmag); % target yaw position\n\nif all(MDs)\n        if xpos > 0    % right loop \n           targetpos = [MDsRy, MDsR, zpos, yawtarg];\n        else\n            targetpos = [MDsLy, MDsL, zpos, yawtarg];\n        end\nelse\n       targetpos = [xtarg, ytarg, zpos, yawtarg];\nend\n\ndelpos = real(targetpos - Pos);"("Pos"=w2586, "m"=w2587, "R"=w2584, "MDs"=w2567, "MDsL"=w2565, "MDsR"=w2566, "MDsLy"="MDsLy", "MDsRy"="MDsRy") -> ("delpos"=w2583:dbl[], "Rotz"=→"Rotz":dbl[][], "targetpos"=→"targetpos":dbl[], "Pos"=→"Pos":dbl[])  [unwired: 1 in, 1 out]
          n868 = local write "upper limit"(dbl[] [0.3, 0.18, -0.65, 6000.0] ("upper limit")) -> ()
          n869 = Replace Array Subset(array=dbl[] [-0.3, -0.18, -0.782, -6000.0] ("lower limit"), new element="lower Z limit", index=2) -> (w2570:dbl[])
          n870 = local write "lower limit"(w2570) -> ()
          n871 = local write "Yaw_tajectory"(TRUE ("Mousetrack_Y")) -> ()
          n872 = local write "Disable Yaw forces"(TRUE ("Mousetrack_Y")) -> ()
          n873 = local write "Disable Y forces"(TRUE ("Disable Y forces")) -> ()
          n874 = local write "Y_trajectory"(TRUE ("Mousetrack_Y")) -> ()
          n875 = local write "Disable -X"(TRUE ("Disable -X")) -> ()
          n876 = local write "deltapos"(w2583) -> ()
          n877 = local write "delpos limits (+/-)\nadmittance control \n(mouse frame)"("delpos limits (+/-)\nadmittance control \nLoop") -> ()
          n878 = local read "Loop time (ms)"() -> (w2585:i64)
          n879 = local read "Loop_L"() -> (w2588:bool)
          n880 = local read "Loop_R"() -> (w2589:bool)
          n881 = local read "Dzone"() -> (w2580:bool)
          n882 = local read "Eight maze on"() -> (w2590:bool)
          n883 = Or(x=w2588, y=w2589) -> (x .or. y?=w2582:bool)
          n884 = Not(x=w2582) -> (.not. x?=w2581:bool)
          n885 = Wait (ms)(milliseconds to wait=w2585) -> ()  [unwired: 1 out]
          n886 = Not(x=w2590) -> (.not. x?=w2592:bool)
          n887 = Or(x=w2580, y=w2581) -> (x .or. y?=w2579:bool)
          n888 = Or(x=w2579, y=w2592) -> (x .or. y?=w2591:bool)
        }
      }
    }
  }
  n889 = while {
    shift-right: ["Joystick control on"] -> _
    shift-left: _ -> [w3117]
    shift-right: [w3110] -> _
    shift-left: _ -> [w3111]
    i -> [w3114]
    stop <- FALSE stop-if-true
    n890 = shared-variable "RT CompactRIO Target\\Mod8\\AI29"() -> (w3120:dbl)  [unwired: 1 in, 1 out]
    n891 = shared-variable "RT CompactRIO Target\\Mod8\\AI23"() -> (w3118:dbl)  [unwired: 1 in, 1 out]
    n892 = shared-variable "RT CompactRIO Target\\Mod8\\AI21"() -> (w3123:dbl)  [unwired: 1 in, 1 out]
    n893 = shared-variable "RT CompactRIO Target\\Mod8\\AI22"() -> (w3122:dbl)  [unwired: 1 in, 1 out]
    n894 = shared-variable "RT CompactRIO Target\\Mod8\\AI30"() -> (w3119:dbl)  [unwired: 1 in, 1 out]
    n895 = shared-variable "RT CompactRIO Target\\Mod8\\AI31"() -> (w3121:dbl)  [unwired: 1 in, 1 out]
    n896 = Less?(x=w3114, y=2) -> (x < y?=w3112:bool)
    n897 = Build Array(w3123, w3122, w3120, w3119, w3118, w3121) -> (w3116:dbl[])
    "Joystick input" <- w3116
    n898 = case shown="True" w3112 {
      tunnel: [w3132 w3133] -> w3110
      tunnel: w3111 -> [w3132 _]
      frame False {
      }
      frame True {
        n899 = flat-sequence {
          tunnel: [w3135] -> w3134
          tunnel: w3134 -> [w3144]
          tunnel: [w3143] -> w3133
          frame #0 {
            n900 = for {
              N: 20 -> [_]
              tunnel: [w3138] -> w3136 mode=indexing
              n901 = shared-variable "RT CompactRIO Target\\Mod8\\AI29"() -> (w3140:dbl)  [unwired: 1 in, 1 out]
              n902 = shared-variable "RT CompactRIO Target\\Mod8\\AI21"() -> (w3142:dbl)  [unwired: 1 in, 1 out]
              n903 = shared-variable "RT CompactRIO Target\\Mod8\\AI22"() -> (w3141:dbl)  [unwired: 1 in, 1 out]
              n904 = shared-variable "RT CompactRIO Target\\Mod8\\AI30"() -> (w3139:dbl)  [unwired: 1 in, 1 out]
              n905 = Build Array(w3142, w3141, w3140, w3139) -> (w3138:dbl[])
            }
            n906 = Transpose 2D Array(2D array=w3136) -> (transposed array=w3135:dbl[][])
          }
          frame #1 {
            n907 = for {
              N: 4 -> [_]
              tunnel: w3144 -> [w3147] mode=indexing
              tunnel: [w3146] -> w3143 mode=indexing
              n908 = call-poly <vilib>:"Mean.vi"("X"=w3147) -> ("mean"=w3146:dbl)  [unwired: 1 out]
            }
          }
        }
      }
    }
    "Jostick offset" <- w3110
    n909 = Array Subset(array=w3116, index=0, length=4) -> (w3128:dbl[])
    n910 = Subtract(x=w3128, y=w3110) -> (x-y=w3127:dbl[])
    n911 = Multiply(x=w3127, y=dbl[] [0.4, 0.4, 0.0, 0.04]) -> (x*y=w3125:dbl[])
    n912 = case shown="False" "Joystick control on" {
      selector: "Joystick control on" -> [w3151 _]
      tunnel: w3125 -> [_ w3154]
      tunnel: w3117 -> [w3150 _]
      frame False {
        n913 = Greater?(x=w3150, y=w3151) -> (0:w3152:bool)
        n914 = case shown="False" w3152 {
          frame False {
          }
          frame True {
            n915 = local write "Manual forces\n(mouse frame)"(dbl[] [0.0, 0.0, 0.0, 0.0]) -> ()
          }
        }
      }
      frame True {
        n916 = local write "Manual forces\n(mouse frame)"(w3154) -> ()
      }
    }
    n917 = case shown="False" "Joystick control on" {
      tunnel: [u32 100 ("Loop time (ms) FDAQ") w3149] -> w3124
      frame False {
      }
      frame True {
        n918 = local read "Loop time (ms)"() -> (w3149:i64)
      }
    }
    n919 = Wait (ms)(milliseconds to wait=w3124) -> ()  [unwired: 1 out]
  }
  n920 = while {
    stop <- FALSE stop-if-true
    n921 = Wait (ms)(milliseconds to wait=u32 10) -> ()  [unwired: 1 out]
    n922 = case shown="True" "Manual \npulse high" {
      tunnel: [FALSE ("DIO0") TRUE ("DIO0")] -> w3156
      frame False {
      }
      frame True {
      }
    }
    n923 = shared-variable "RT CompactRIO Target\\Mod7\\DIO0"(w3156) -> ()  [unwired: 1 in, 1 out]
    n924 = local write "SynPulseOn"(w3156) -> ()
  }
  n925 = while {
    shift-right: ["Close file and open new file"] -> _
    shift-left: _ -> [w3167]
    stop <- FALSE stop-if-true
    n926 = Wait (ms)(milliseconds to wait=u32 100) -> ()  [unwired: 1 out]
    n927 = Greater?(x="Close file and open new file", y=w3167) -> (0:w3165:bool)
    n928 = case shown="True" w3165 {
      tunnel: [FALSE TRUE] -> w3164
      frame False {
      }
      frame True {
        n929 = local write "Close file and open new file"(FALSE ("Close file and open new file")) -> ()
      }
    }
    n930 = Or(x=w3164, y="Stop raspberry pi") -> (x .or. y?=w3162:bool)
    n931 = shared-variable "RT CompactRIO Target\\Mod6\\DIO12"("Record to current file") -> ()  [unwired: 1 in, 1 out]
    n932 = shared-variable "RT CompactRIO Target\\Mod6\\DIO10"("Stop raspberry pi") -> ()  [unwired: 1 in, 1 out]
    n933 = shared-variable "RT CompactRIO Target\\Mod6\\DIO11"(w3162) -> ()  [unwired: 1 in, 1 out]
  }
  n934 = while {
    stop <- FALSE stop-if-true
    n935 = flat-sequence {
      tunnel: [w3209] -> w3173
      tunnel: w3173 -> [w3708]
      frame #0 {
        n936 = Wait (ms)(milliseconds to wait=u32 250) -> ()  [unwired: 1 out]
      }
      frame #1 {
        n937 = while {
          stop <- w3176 stop-if-true
          n938 = local read "Loop_R Exit"() -> (w3177:bool)
          n939 = local read "Loop_L Exit"() -> (w3178:bool)
          n940 = Wait (ms)(milliseconds to wait=u32 250) -> ()  [unwired: 1 out]
          n941 = Or(x=w3178, y=w3177) -> (x .or. y?=w3176:bool)
        }
      }
      frame #2 {
        n942 = local read "Loop_L Exit"() -> (w3180:bool)
        n943 = case shown="True" w3180 {
          frame False {
            n944 = while {
              stop <- w3185 stop-if-true
              n945 = local read "op-space pos\n(global frame)"() -> (w3184:dbl[])
              n946 = local read "exit_pos"() -> (w3183:dbl[])
              n947 = Wait (ms)(milliseconds to wait=u32 10) -> ()  [unwired: 1 out]
              n948 = Index Array(array=w3183, index=0) -> (element=w3182:dbl)
              n949 = Negate(x=w3182) -> (-x=w3181:dbl)
              n950 = Index Array(array=w3184, index=1) -> (element=w3190:dbl)
              n951 = Index Array(array=w3184, index=0) -> (element=w3191:dbl)
              n952 = Less?(x=w3190, y=0.0) -> (x < y?=w3187:bool)
              n953 = Less?(x=w3191, y=w3181) -> (x < y?=w3188:bool)
              n954 = And(x=w3188, y=w3187) -> (x .and. y?=w3185:bool)
            }
          }
          frame True {
            n955 = while {
              stop <- w3196 stop-if-true
              n956 = local read "op-space pos\n(global frame)"() -> (w3207:dbl[])
              n957 = local read "exit_pos"() -> (w3206:dbl[])
              n958 = Wait (ms)(milliseconds to wait=u32 10) -> ()  [unwired: 1 out]
              n959 = Index Array(array=w3207, index=1) -> (element=w3200:dbl)
              n960 = Index Array(array=w3206, index=0) -> (element=w3201:dbl)
              n961 = Index Array(array=w3207, index=0) -> (element=w3202:dbl)
              n962 = Less?(x=w3200, y=0.0) -> (x < y?=w3197:bool)
              n963 = Greater?(x=w3202, y=w3201) -> (0:w3198:bool)
              n964 = And(x=w3198, y=w3197) -> (x .and. y?=w3196:bool)
            }
          }
        }
      }
      frame #3 {
        n965 = local write "Eight maze on"(FALSE ("Eight maze on")) -> ()
      }
      frame #4 {
        n966 = while {
          tunnel: [w3214] -> w3209
          stop <- w3216 stop-if-true
          n967 = local read "Loop_L Exit"() -> (w3223:bool)
          n968 = local write "Disable Yaw forces"(TRUE ("Disable Yaw forces")) -> ()
          n969 = local write "Disable Y forces"(TRUE ("Disable Y forces")) -> ()
          n970 = local write "Disable -X"(TRUE ("Disable -X")) -> ()
          n971 = local write "delpos limits (+/-)\nadmittance control \n(mouse frame)"(dbl[] [0.0002, 0.0002, 0.0, 0.01] ("delpos limits (+/-)\nadmittance control \nDzone")) -> ()
          n972 = local read "exit_cen"() -> (w3228:dbl[])
          n973 = local read "op-space pos\n(global frame)"() -> (w3222:dbl[])
          n974 = local read "op-space pos\n(global frame)"() -> (w3214:dbl[])
          n975 = local read "exit_cen"() -> (w3218:dbl[])
          n976 = local read "Rexit"() -> (w3227:dbl)
          n977 = mathscript code="xpos = Pos(1,1);\nypos = Pos(1,2);\nzpos = Pos(1,3);\nyawpos = Pos(1,4);\n\nRotz = [cos(yawpos),-sin(yawpos),0; sin(yawpos),cos(yawpos),0; 0,0,1];\nxhat = [1, 0, 0]';\nzhat = [0, 0, 1]';\n\nif all(Lexit)\n       RLsgn = 1;\nelse\n        RLsgn = -1\nend\n w_cen(1) = RLsgn*w_cen(1);        % center on other side of x=0 if Rloop exit\n\n       xcen = xpos - w_cen(1);\n       ycen = ypos - w_cen(2);\n       Rmag = real((xcen^2 + ycen^2)^0.5);\n       xtarg = R/Rmag*xcen  + w_cen(1);\n       ytarg = R/Rmag*ycen + w_cen(2);      \n\nvecpos = [xcen, ycen, 0]';         % position vector, zero'd circle\nvecyaw = RLsgn*cross(vecpos,zhat);  % yaw vector\nvecyaw_o = Rotz'*vecyaw;        %  yaw vector transformed by actual yaw\nyawerrsign = sign(0 - vecyaw_o(2));  % sign of yaw error\nyawerrmag = acos(dot(vecyaw_o,xhat)/(norm(vecyaw_o)*norm(xhat))); % magnitude of yaw error   \nyawtarg  = yawpos - yawerrsign*real(yawerrmag); % target yaw position\n\ntargetpos = [xtarg, ytarg, zpos, yawtarg];\n\ndelpos = real(targetpos - Pos);"("Pos"=w3214, "R"=w3227, "w_cen"=w3228, "Lexit"=w3223) -> ("delpos"=w3215:dbl[], "w_cen"=→"w_cen 2":dbl[], "Rmag"=→"Rmag":dbl)  [unwired: 1 in, 1 out]
          n978 = Index Array(array=w3222, index=1) -> (element=w3220:dbl)
          n979 = Index Array(array=w3218, index=1) -> (element=w3217:dbl)
          n980 = Less?(x=w3220, y=w3217) -> (x < y?=w3216:bool)
          n981 = local write "deltapos"(w3215) -> ()
          n982 = Wait (ms)(milliseconds to wait=u32 10) -> ()  [unwired: 1 out]
        }
      }
      frame #5 {
        n983 = while {
          tunnel: w3708 -> [w3723]
          stop <- w3716 stop-if-true
          n984 = local read "op-space pos\n(global frame)"() -> (w3719:dbl[])
          n985 = local write "Disable Yaw forces"(TRUE ("Disable Yaw forces")) -> ()
          n986 = local write "Disable Y forces"(TRUE ("Disable Y forces")) -> ()
          n987 = local read "op-space pos\n(global frame)"() -> (w3722:dbl[])
          n988 = local write "Disable -X"(TRUE ("Disable -X")) -> ()
          n989 = local write "upper limit"(dbl[] [0.3, 0.18, -0.65, 6000.0] ("upper limit")) -> ()
          n990 = local write "lower limit"(dbl[] [-0.3, -0.34, -0.782, -6000.0] ("lower limit")) -> ()
          n991 = Index Array(array=w3719, index=1) -> (element=w3718:dbl)
          n992 = Less?(x=w3718, y="Mouse YStop") -> (x < y?=w3716:bool)
          n993 = local write "delpos limits (+/-)\nadmittance control \n(mouse frame)"(dbl[] [0.0004, 0.0002, 0.0, 0.01] ("delpos limits (+/-)\nadmittance control \nLoop")) -> ()
          n994 = Index Array(array=w3723, index=3) -> (element=w3724:dbl)
          n995 = mathscript code="xpos = Pos(1,1);\nypos = Pos(1,2);\nzpos = Pos(1,3);\nyawpos = Pos(1,4);\n\nyawtarg = real(round((yaw_init)/(pi/2))*pi/2);\n\nxtarg = 0;\n\ntargetpos = [xtarg, ypos, zpos, yawtarg];\n\ndelpos = real(targetpos - Pos);"("yaw_init"=w3724, "Pos"=w3722) -> ("delpos"=w3721:dbl[])  [unwired: 1 in, 1 out]
          n996 = local write "deltapos"(w3721) -> ()
          n997 = Wait (ms)(milliseconds to wait=u32 10) -> ()  [unwired: 1 out]
        }
      }
      frame #6 {
        n998 = local write "Manual position control"(TRUE ("Manual position control")) -> ()
        n999 = local write "End Wheel"(FALSE ("End Wheel")) -> ()
      }
      frame #7 {
        n1000 = while {
          stop <- FALSE stop-if-true
          n1001 = Wait (ms)(milliseconds to wait=u32 50) -> ()  [unwired: 1 out]
        }
      }
    }
  }
  n1002 = flat-sequence "Exit sequence latched switch" {
    frame #0 {
      n1003 = local write "End Wheel"(FALSE ("End Wheel")) -> ()
      n1004 = local write "Loop_R Exit"(FALSE ("Loop_R Exit")) -> ()
      n1005 = local write "Loop_L Exit"(FALSE ("Loop_L Exit")) -> ()
    }
    frame #1 {
      n1006 = while {
        stop <- w3882 stop-if-true
        n1007 = local read "Eight maze on"() -> (w3884:bool)
        n1008 = local read "End Wheel"() -> (w3883:bool)
        n1009 = local read "Dzone"() -> (w3881:bool)
        n1010 = Wait (ms)(milliseconds to wait=u32 250) -> ()  [unwired: 1 out]
        n1011 = Not(x=w3881) -> (.not. x?=w3880:bool)
        n1012 = Compound Arithmetic op=AND(w3883, w3884, w3880) -> (w3882:bool)
      }
    }
    frame #2 {
      n1013 = local read "Loop_L"() -> (→"Loop_L Exit":bool)
      n1014 = local read "Loop_R"() -> (→"Loop_R Exit":bool)
      n1015 = local write "Begin Wheel"(FALSE ("Begin Wheel")) -> ()
    }
    frame #3 {
      n1016 = while {
        stop <- FALSE stop-if-true
        n1017 = Wait (ms)(milliseconds to wait=u32 250) -> ()  [unwired: 1 out]
      }
    }
  }
  n1018 = while {
    stop <- FALSE stop-if-true
    n1019 = Wait (ms)(milliseconds to wait=u32 250) -> ()  [unwired: 1 out]
    n1020 = shared-variable "RT CompactRIO Target\\Mod1\\DI2"() -> (w3898:bool)  [unwired: 1 in, 1 out]
    n1021 = shared-variable "RT CompactRIO Target\\Mod1\\DI3"() -> (w3897:bool)  [unwired: 1 in, 1 out]
    n1022 = shared-variable "RT CompactRIO Target\\Mod1\\DI0"() -> (w3900:bool)  [unwired: 1 in, 1 out]
    n1023 = shared-variable "RT CompactRIO Target\\Mod1\\DI1"() -> (w3899:bool)  [unwired: 1 in, 1 out]
    n1024 = Not(x=w3898) -> (.not. x?=w3902:bool)
    n1025 = Not(x=w3897) -> (.not. x?=w3901:bool)
    n1026 = Not(x=w3900) -> (.not. x?=w3904:bool)
    n1027 = Not(x=w3899) -> (.not. x?=w3903:bool)
    n1028 = shared-variable "RT CompactRIO Target\\Mod6\\DIO2"(w3902) -> ()  [unwired: 1 in, 1 out]
    n1029 = shared-variable "RT CompactRIO Target\\Mod6\\DIO3"(w3901) -> ()  [unwired: 1 in, 1 out]
    n1030 = shared-variable "RT CompactRIO Target\\Mod1\\DO2"(w3898) -> ()  [unwired: 1 in, 1 out]
    n1031 = shared-variable "RT CompactRIO Target\\Mod1\\DO3"(w3897) -> ()  [unwired: 1 in, 1 out]
    n1032 = shared-variable "RT CompactRIO Target\\Mod6\\DIO0"(w3904) -> ()  [unwired: 1 in, 1 out]
    n1033 = shared-variable "RT CompactRIO Target\\Mod6\\DIO1"(w3903) -> ()  [unwired: 1 in, 1 out]
    n1034 = shared-variable "RT CompactRIO Target\\Mod1\\DO0"(w3900) -> ()  [unwired: 1 in, 1 out]
    n1035 = shared-variable "RT CompactRIO Target\\Mod1\\DO1"(w3899) -> ()  [unwired: 1 in, 1 out]
    n1036 = shared-variable "RT CompactRIO Target\\Mod2\\DI2"() -> (w3892:bool)  [unwired: 1 in, 1 out]
    n1037 = shared-variable "RT CompactRIO Target\\Mod2\\DI3"() -> (w3891:bool)  [unwired: 1 in, 1 out]
    n1038 = shared-variable "RT CompactRIO Target\\Mod2\\DI0"() -> (w3894:bool)  [unwired: 1 in, 1 out]
    n1039 = shared-variable "RT CompactRIO Target\\Mod2\\DI1"() -> (w3893:bool)  [unwired: 1 in, 1 out]
    n1040 = shared-variable "RT CompactRIO Target\\Mod2\\DO2"(w3892) -> ()  [unwired: 1 in, 1 out]
    n1041 = shared-variable "RT CompactRIO Target\\Mod2\\DO3"(w3891) -> ()  [unwired: 1 in, 1 out]
    n1042 = shared-variable "RT CompactRIO Target\\Mod2\\DO0"(w3894) -> ()  [unwired: 1 in, 1 out]
    n1043 = shared-variable "RT CompactRIO Target\\Mod2\\DO1"(w3893) -> ()  [unwired: 1 in, 1 out]
    n1044 = case shown="True" w3894 {
      tunnel: w3893 -> [_ w3906]
      tunnel: w3891 -> [_ w3905]
      frame False {
      }
      frame True {
        n1045 = local write "Manual position control"(w3906) -> ()
        n1046 = local write "End Wheel"(w3905) -> ()
      }
    }
  }
